vi "Dashboard Main.vi"() -> ()   [LabVIEW 2018]
uses:
  <vilib>/Utility/miscctls.llb/LVRowAndColumnTypeDef.ctl
  <vilib>/event_ctls.llb/eventvkey.ctl
  <vilib>/Utility/xml.llb/Read From XML File(array).vi
  <vilib>/Utility/xml.llb/Write to XML File(string).vi
  <vilib>/Rock Robotics/Network Tables/NT Read Boolean.vi
  <vilib>/Rock Robotics/Network Tables/NT Write Boolean.vi
  <vilib>/Rock Robotics/WPI/Dashboard/WPI_DashboardLogging Global.vi
  <vilib>/vision/NI_Vision_Development_Module.lvlib
panel:
  in  "TCP":refnum<k5>
  in  "Rec Mode":enum32{"Stop", "Record", "Playback"}(radio)
  out "Image Message":string="Timeout in Camera Communications"
  in  "Dashboard Tab":T1(tab)=enum."TeleOp"
  in  "CheckList":i32(listbox)
  in  "Driver Profile":u16(ring) items=["N/A"]
  in  "Camera Name":string(combo)="limelight"
  in  "Camera Settings":T2={"Frame Rate"=20, "Compression"=60, "Size"=1, "DB Camera Config"=FALSE} {"Size" items=["640x480", "320x240", "160x120"]}
  in  "Warning Time (s)":dbl=30.0
  out "Pressure_Leak":bool
  out "Ret_CARGO Right":bool
  out "Ret_HATCH Right":bool
  out "Ret_CARGO Left":bool
  out "Ret_HATCH Left":bool
  out "Ret_CARGO Center":bool
  out "Elevator_Motor_Failure_2":bool
  out "Elevator_Stall":bool
  out "Range_Color_Front-Right":u32(colorbox)
  in  "Right":bool
  in  "Reticule":T3(ring)
  in  "Save":bool
  in  "Up":bool
  in  "Down":bool
  in  "Left":bool
  out "Out_Of_Time":bool caption="Mode_Butterfly"
  out "Match Time(s)":sgl
  out "Intake_In":bool caption="Mode_Butterfly"
  in  "Climb_Safety":bool
  out "Master_Caution":bool caption="Mode_Butterfly"
  out "Climb_Sequence":string
  out "Range_to_Target (R)":i16(slide)=-100 scale=-10.0..-50.0
  out "Range_to_Target (L)":i16(slide)=-100 scale=-50.0..-10.0
  out "Tilt_Interlock":bool
  out "Battery_Critical":bool
  out "Battery_Voltage":dbl(slide) scale=11.0..13.0
  out "COM_Warning":bool
  out "Elevator_Moving":bool caption="Mode_Butterfly"
  out "Range_Color_Back":u32(colorbox)
  out "Range_Color_Front-Left":u32(colorbox)
  out "Range_Color_Right":u32(colorbox)
  out "Range_Color_Left":u32(colorbox)
  out "Hatch_Ship_Light":bool
  out "Hatch_Rocket_1_Light":bool
  out "Hatch_Ground_Light":bool
  out "Hatch_Feeder_Light":bool
  out "Hatch_Rocket_2_Light":bool
  out "Hatch_Rocket_3_Light":bool
  out "Pressure_Visualize":dbl(slide) scale=0.0..120.0
  out "Autopilot":bool caption="Mode_Butterfly"
  in  "Master_Safety_Override_1":bool
  in  "Master_Safety_Override_2":bool
  out "Climb_Light":bool
  out "At Climb_Height":bool caption="Mode_Butterfly"
  out "PTO_Engaged":bool caption="Mode_Butterfly"
  in  "Climb":bool
  out "Mode_Butterfly":bool
  out "Compressor_On":bool
  out "Hatch_Ejection_State":bool caption="Mode_Butterfly"
  out "Elevator_Brake_State":bool
  out "Mode_Shift":bool caption="Mode_Butterfly"
  out "Capture_Cargo":bool caption="Mode_Butterfly"
  out "Capture_Hatch":bool caption="Mode_Butterfly"
  in  "Hatch_Ground":bool
  in  "Hatch_Feeder":bool
  in  "Hatch_Rocket_2":bool
  in  "Hatch_Rocket_1":bool
  in  "Hatch_Ship":bool
  in  "Hatch_Rocket_3":bool
  out "Elevator_Stow_Light":bool
  in  "Elevator_Stow":bool
  out "Cargo_Ground_Light":bool
  out "Cargo_Feeder_Light":bool
  out "Cargo_Ship_Light":bool
  out "Cargo_Rocket_3_Light":bool
  in  "Cargo_Ground":bool
  in  "Cargo_Feeder":bool
  out "Cargo_Rocket_2_Light":bool
  out "Cargo_Rocket_1_Light":bool
  in  "Cargo_Ship":bool
  in  "Cargo_Rocket_1":bool
  in  "Cargo_Rocket_2":bool
  in  "Cargo_Rocket_3":bool
  out "State_Conflict":bool caption="Mode_Butterfly"
  out "Combined Camera Feed":T4(plugin-control)
  out "Elevator_Pos_Visual":dbl(slide) scale=34.5..89.0
  in  "Vision_Target_L_R":bool
  out "Elevator_Goal_Visual":dbl(slide) scale=34.5..89.0
  out "Elevator_Power":dbl(knob) scale=-1.0..1.0
  in  "Climb_Level":u8(slide)=1 scale=0.0..2.0
  out "E1 Warning":bool
  out "E2 Warning":bool
  out "E3 Warning":bool
  out "Elevator_3_Current":dbl format="%.1g"
  out "Elevator_2_Current":dbl format="%.1g"
  out "Elevator_1_Current":dbl format="%.1g"
  out "Slow_Loop":bool
  in  "Elevator_Kf_1":dbl(slide)=0.2 min=0.0 max=1.0 scale=0.0..1.0
  in  "Elevator_Kf_2":dbl(slide)=0.2 min=0.0 max=1.0 scale=0.0..1.0
  in  "Elevator_Kf_3":dbl(slide) min=0.0 max=1.0 scale=0.0..1.0
  in  "Select Auto":string(combo)="Select Autonomous ..."
  out "Camera Perf":string
  in  "Elevator_Kf_Climb":dbl(slide)=0.1 min=0.0 max=1.0 scale=0.0..1.0
  out "Control Loop Time (ms)":u32
  in  "Vacuum_Pump":dbl(slide)=0.6 min=0.0 max=1.0 scale=0.0..1.0
  out "Range_Right":dbl format="%.1g"
  in  "Elevator_Manual":bool
  in  "Drive_Encoder_Reset":bool
  out "Right_Drive_Pos":dbl
  out "Left_Drive_Pos":dbl
  out "Range_Left":dbl format="%.1g"
  out "Range_Front-Left":dbl format="%.1g"
  out "Range_Front-Right":dbl format="%.1g"
  out "Left_Drive_Vel":dbl format="%.1g"
  out "Right_Drive_Vel":dbl format="%.1g"
  out "Elevator_Pos":dbl format="%.1g"
  out "Range_Back":dbl
  out "Tank_Pressure":dbl format="%.1f"
  in  "Super_Test_Mode":bool
  out "Ground_Height":dbl format="%.1g"
  in  "Overclock":bool=TRUE
  in  "Reinit_Stow_Vacuum":bool
  in  "LimeLight_Override":bool
  out "Elevator_Encoder_Malfunction":bool
  out "Elevator_Motor_Failure":bool
  out "Robot_On_Ground":bool=TRUE
  out "Robot_Off_Ground":bool
  out "Check_Limit_Switch":bool
  in  "Tilt_Safety_Override":bool
  in  "Defense_Driving":bool
  out "Combined Error String":string
  out "NT Connection":bool
  out "Mode":T5(ring)=enum."Auto Disabled"
  in  "Test Slider":dbl(slide) scale=0.0..100.0 scale format="%#_3g"
  in  "On/Off":bool caption="Solenoid"
  in  "Test Name":u16(ring) items=["Select the test to run..."]
  in  "Test Tree":string(tree)
  in  "Motor":cluster{"Value":dbl, "Enable":bool} {"Value" scale=-1.0..1.0 scale format="%#_3g"}
  out "Progress":T6 {"Test Progress" scale=0.0..100.0}
  in  "Rev/Fwd":cluster{"Forward":bool, "Reverse":bool}
  in  "Test Ring":u16(ring) items=["Monochrome", "Color"]
  out "Cmd Status":string
  in  "Execute Command":bool
  in  "Command Params":string[][](table)
  in  "Command Selection":i32(listbox)
  out "Tree":string(tree)
  out "Background":bool
  # "Camera Selection"
  # "Match End Warning (s)"
  # "Camera Settings"
  # "89.0"
  # "11"
  # "13"
  # "120"
  # "0"
  # "Valkyrie"
  # "B"
  # "3"
  # "2"
  # "0"
  # "34.5"
  # "Control Loop (ms)"
  # "Elevator Feed Forward Coefficients"
  # "Drive Wheel Velocities (ft/s)"
  # "Manual Elevator Override"
  # "Tilt Interlock Off"
  # "Wide-Cam Override"
  # "Reinit.  Vacuum in Stow"
  # "Super Test Mode"
  # "Elevator Position (in)"
  # "Prox Sensors (in)"
  # "Auto Elevator"
  # "Safe"
  # "Vacuum \nPump Power"
  # "Normal"
  # "Normal"
  # "Safe"
  # "Stage 2"
  # "Stage 3"
  # "Climb"
  # "Ground Height (in)"
  # "Elevator Motor Currents (A)"
  # "On \nGround"
  # "Off\nGround"
  # "E1"
  # "E2"
  # "E3"
  # "Tank Pressure (psi)"
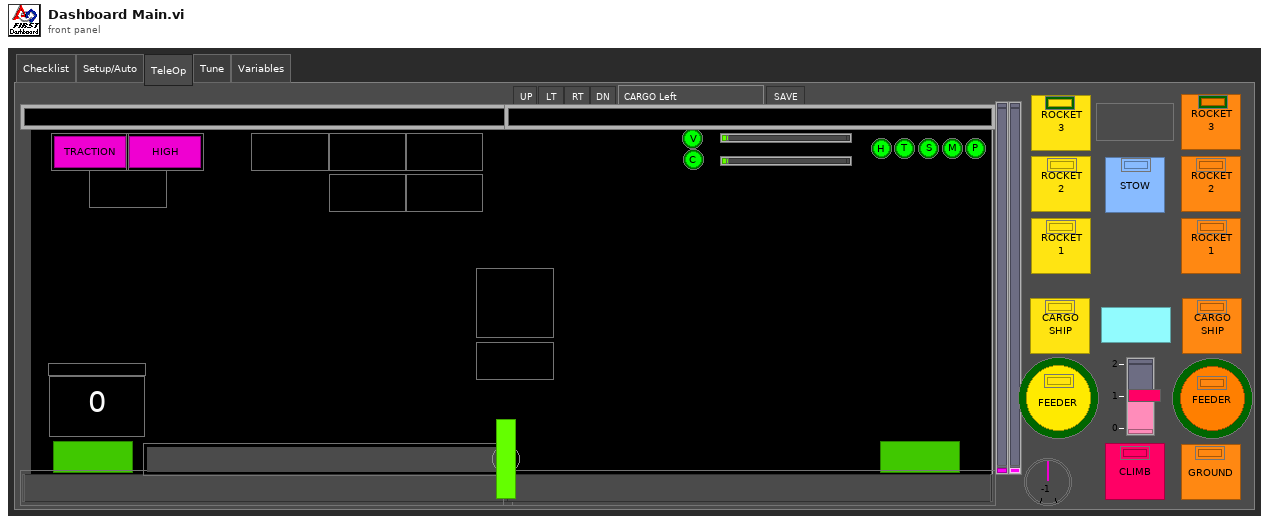
[diagram p1: front panel]
types:
  T1 = enum32{"Checklist", "Setup/Auto", "TeleOp", "Tune", "NT", "Test", "Commands", "Variables"}
  T2 = cluster{"Frame Rate":i32, "Compression":i32, "Size":u16, "DB Camera Config":bool}
  T3 = enum16{"CARGO Left", "CARGO Right", "HATCH Left", "HATCH Right", "CARGO Center"}
  T4 = typedef "IMAQ Image.ctl" = refnum<image>
  T5 = enum8{"Tele-Op Disabled", "Tele-Op Enabled", "Auto Disabled", "Auto Enabled", "Test Disabled", "Test Enabled", "Disconnected", "No Code", "E-Stop"}
  T6 = cluster{"Test Progress":u8, "Test Progress Text":string}
  T7 = cluster{"Save Path":path, "Interval (s)":dbl, "Keep":i32}
  T8 = enum32{"Drive", "Camera", "Basic", "Custom", "Test", "Commands", "Checklist", "Variables"}
  T9 = cluster{"IDs":cluster{"RPC field ID":u16, "Unique ID":u16}, "String":string}
  T10 = typedef "Image Type" = u32
  T11 = cluster{"Camera Name":string, string, "Saved DB Images Info":cluster{"Save Path":path, "Interval (s)":dbl, "Keep":i32}}
  T12 = cluster{"Ret_CARGO Left":refnum<vi>, "Ret_CARGO Right":refnum<vi>, "Ret_HATCH Left":refnum<vi>, "Ret_HATCH Right":refnum<vi>, "Ret_CARGO Center":refnum<vi>}
  T13 = enum32{"Checklist", "-", "TeleOp", "Tune", "NT", "Test", "Commands", "Variables"}
  T14 = cluster{"Error Strings":string, "Disable Counts":cluster{u16, u16}, "Rail Faults":cluster{u16, u16, u16}, "Robot IP":string, "DB Mode":u8, "Event Info":cluster{"Name":string, "Type":u8, "Number":u16, "Replay":u8}}
  T15 = cluster{"Storage":cluster{"Disk Free":u64, "RAM Block":u32, "RAM free":u32}, "CPU Utilization":cluster{"CPU % ISR":sgl, "CPU % Time Crit":sgl, "CPU % Timed Str":sgl, "CPU % High":sgl, "CPU % Above":sgl, "CPU % Normal":sgl, "CPU % Low":sgl}, "CAN":cluster{"% Bus Utilization":sgl, "Bus Off Cnt":u32, "TX_FIFO Full Cnt":u32, "Receive Error Cnt":u8, "Transmit Error Cnt":u8}, "HID":cluster{"HID Outputs":u32, "Rumble Low":u16, "Rumble High":u16}[]}
  T16 = cluster{"Status bits":cluster{"Test Mode":bool, "Autonomous":bool, "Enabled":bool, "Code Start":bool, "Brownout":bool, "Reserved 2":bool, "Reserved 3":bool, "E-Stop":bool}, "Code Trace":cluster{"Disabled":bool, "TeleOp":bool, "Auto":bool, "Test":bool}, "Controller Type":enum16{"unknown", "cRIO", "roboRio"}, "Code?":enum16{"unknown", "noCode", "code"}, "Battery V":dbl}
  T17 = cluster{"Control Bits":cluster{"TestMode":bool, "Autonomous":bool, "Enabled":bool, "FMS Present":bool, bool, bool, bool, "E-Stop":bool}, "Team Station ":u8, "Countdown":sgl, "Joystick Values":cluster{"Axes":dbl[], "Buttons":bool[], "POVs":i16[]}[]}
  T18 = cluster{"Operation":enum16{"Update", "Clear"}, "Color Box":u32}[]
  T19 = typedef "eventvkey.ctl" = enum16{"ASCII", "Enter", "Return", "Shift", "Ctrl", "Alt", "Cmd", "Opt", "Caps", "NumLock", "Clear", "Break", "Up", "Down", "Left", "Right", "Insert", "Delete", "Home", "End", "PageUp", "PageDown", "Escape", "Help", "Pause", "ScrollLock", "F1", "F2", "F3", "F4", "F5", "F6", "F7", "F8", "F9", "F10", "F11", "F12", "F13", "F14", "F15", "F16", "F17", "F18", "F19", "F20", "F21", "F22", "F23", "F24", "Play", "VolumeUp", "VolumeDown", "Mute", "Two Byte Char"}
  T20 = cluster{"Image Size":bool, "Image Type":bool, "Pixel Value":bool, "ROI Information":bool, "Zoom Factor":bool}
  T21 = cluster{"Operation":enum16{"Update", "Clear"}, "Color Box":u32}
  T22 = typedef "LVRowAndColumnTypeDef.ctl" = cluster{"Row":i32, "Column":i32}
  T23 = cluster{"Shift":bool, "Ctrl":bool, "Alt":bool, "Cmd":bool, "Opt":bool}
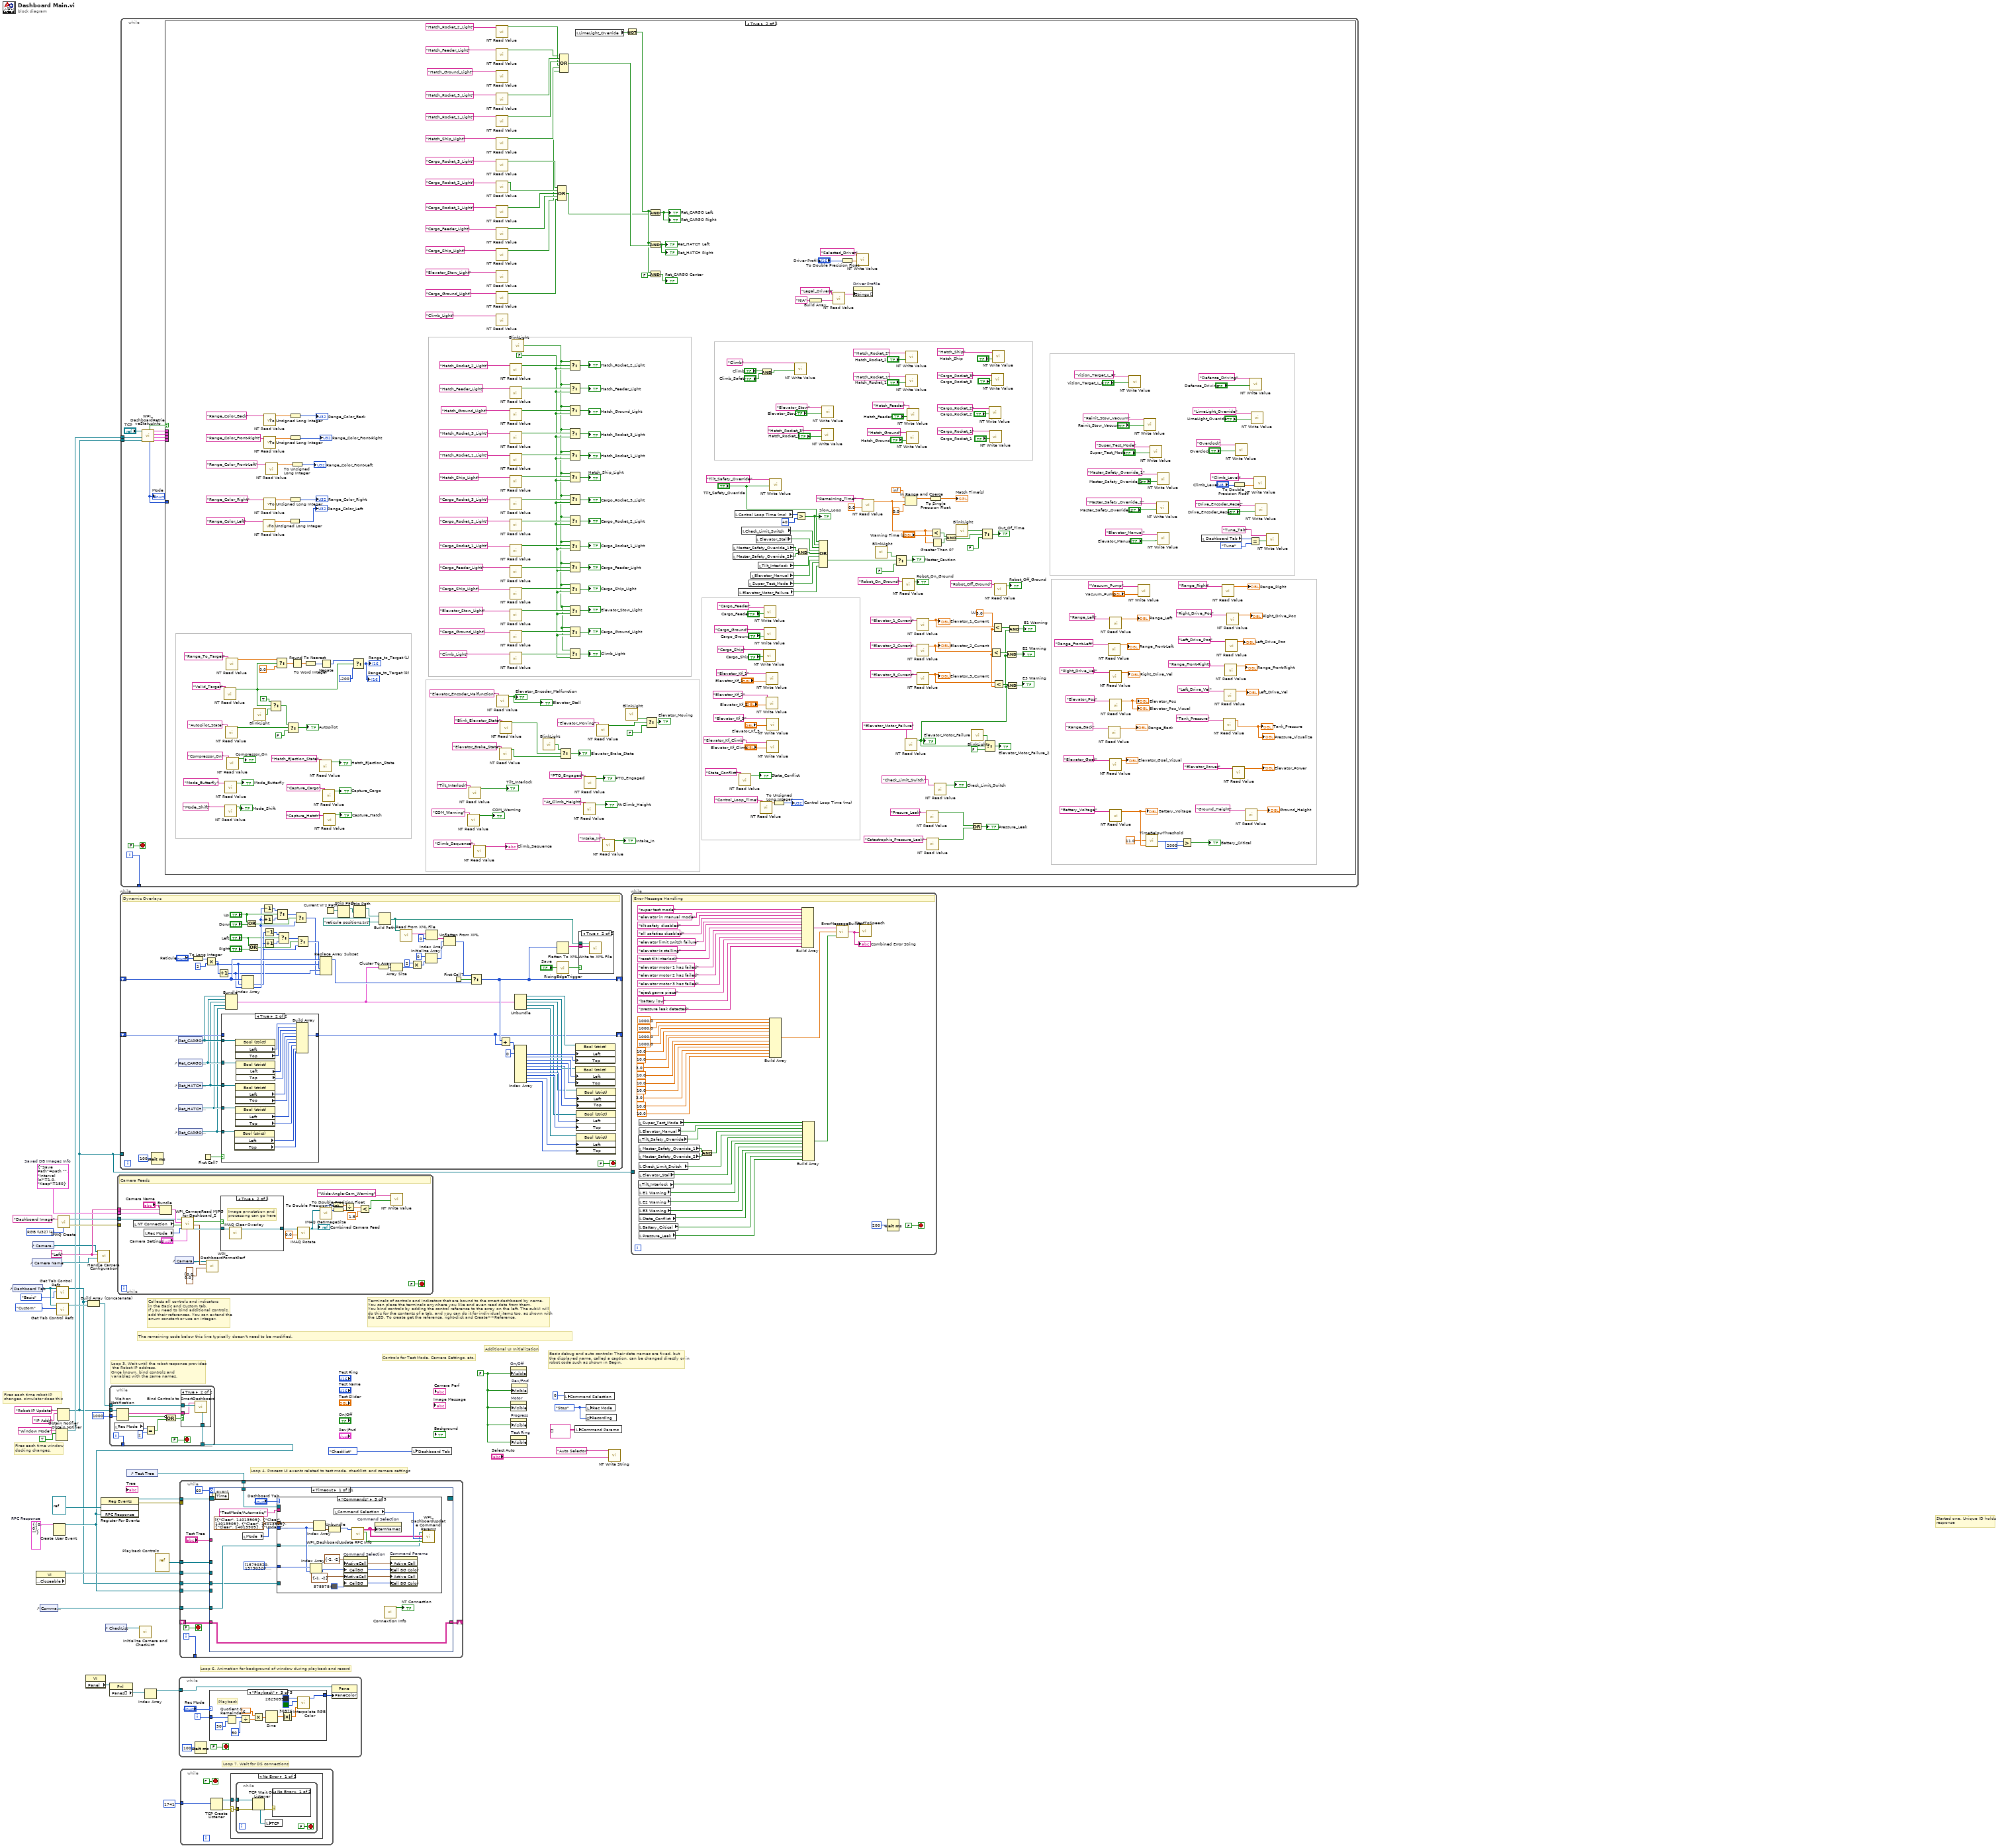
[diagram p0: block diagram]
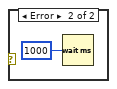
[diagram p4: hidden frame]
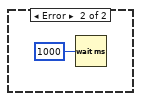
[diagram p5: hidden frame]
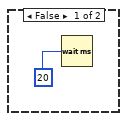
[diagram p6: hidden frame]
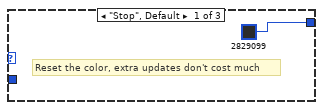
[diagram p7: hidden frame]
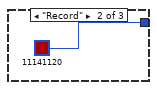
[diagram p8: hidden frame]
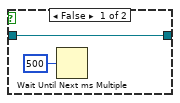
[diagram p10: hidden frame]
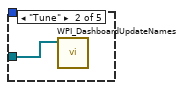
[diagram p12: hidden frame]
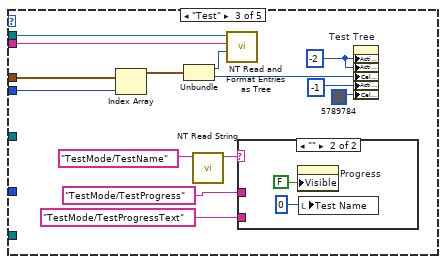
[diagram p13: hidden frame]
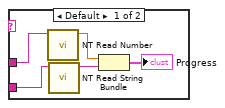
[diagram p14: hidden frame]
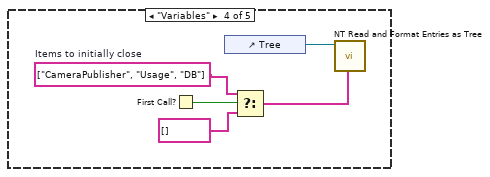
[diagram p15: hidden frame]
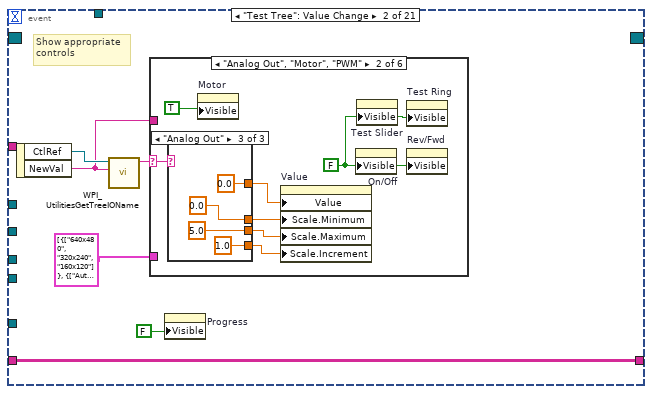
[diagram p16: hidden frame]
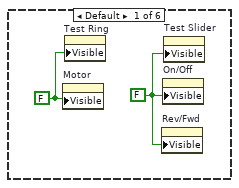
[diagram p17: hidden frame]
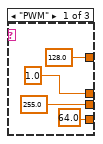
[diagram p18: hidden frame]
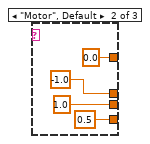
[diagram p19: hidden frame]
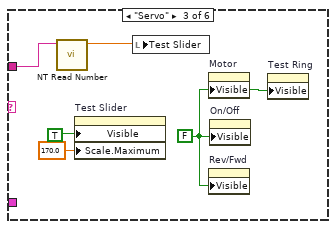
[diagram p20: hidden frame]
diagram:
  w4 = T7 {"Save Path"=path "", "Interval (s)"=1.0, "Keep"=180}  # Saved DB Images Info
  w3 = "Left"
  w15 = T9 {"IDs"={"RPC field ID"=0, "Unique ID"=0}, "String"=""}  # RPC Response
  w25 = enum32{"Stop", "Record", "Playback"}."Stop" ("Rec Mode")
  w19 = FALSE ("Visible")
  w42 = T10 4 items=["Grayscale (U8)", "Grayscale (I16)", "Grayscale (SGL)", "Complex (CSG)", "RGB (U32)", "HSL (U32)", "RGB (U64)"] ("Image Type")
  # "Started one, Unique ID holds\nresponse"
  # "Loop 7. Wait for DS connections"
  # "Basic debug and auto controls: Their data names are fixed, but\nthe displayed name, called a caption, can be changed directly or in\nrobot code such as shown in Begin."
  # "Controls for Test Mode, Camera Settings, etc."
  # "Additional UI Initialization"
  # "Loop 6. Animation for background of window during playback and record"
  # "Fires each time robot IP\nchanges, simulator does this"
  # "Fires each time window\ndocking changes."
  # "Collects all controls and indicators\nin the Basic and Custom tab.\nIf you need to bind additional controls,\nadd their references. You can extend the\nenum constant or use an integer."
  # "The remaining code below this line typically doesn't need to be modified."
  # "Loop 4. Process UI events related to test mode, checklist, and camera settings"
  # "Terminals of controls and indicators that are bound to the smart dashboard by name.\nYou can place the terminals anywhere you like and even read data from them.\nYou bind controls by adding the control reference to the array on the left. The subVI will\ndo this for the contents of a tab, and you can do it for individual items too, as shown with\nthe LED. To create get the reference, right-click and Create>>Reference."
  # "Loop 3. Wait until the robot response provides\n the Robot IP address.\nOnce known, bind controls and\nvariables with the same names."
  n1 = control-ref of="Dashboard Tab"() -> (w23:refnum<vi>)
  n2 = control-ref of="Camera Name"() -> (w10:refnum<vi>)
  n3 = control-ref of="Camera Settings"() -> (w2:refnum<vi>)
  n4 = property class="VI" props=["Front Panel.Closeable"]() -> (reference out=w24:refnum<vi>)  [unwired: 2 in, 2 out]
  n5 = control-ref of="Command Params"() -> (w11:refnum<vi>)
  n6 = Create User Event(user event datatype=w15) -> (user event=w12:refnum<user-event>)  [unwired: 1 in, 1 out]
  n7 = Obtain Notifier(name (unnamed)="Window Mode", notification data type=TRUE) -> (notifier out=w18:refnum<notifier>)  [unwired: 2 in, 2 out]
  n8 = call <vilib>:"Get Tab Control Refs.vi"("Page Index"=T8."Basic" ("Dashboard Tab"), "TabControl in"=w23) -> ("ControlsOnPage"=w9:refnum<vi>[])  [unwired: 9 in]
  n9 = call <vilib>:"Get Tab Control Refs.vi"("Page Index"=T8."Custom" ("Dashboard Tab"), "TabControl in"=w23) -> ("ControlsOnPage"=w22:refnum<vi>[])  [unwired: 9 in]
  n10 = Obtain Notifier(name (unnamed)="Robot IP Update", notification data type="IP Addr" ("name (unnamed)")) -> (notifier out=w1:refnum<notifier>)  [unwired: 2 in, 2 out]
  n11 = call "IMAQ Create"("Image Name"="Dashboard Image", "Image Type"=w42) -> ("New Image"=w40:T4, "error out"=w39:errorcluster)  [unwired: 2 in, 1 out]
  n12 = property class="VI"() -> ("Panel"=w32:refnum<vi>)  [unwired: 2 in, 2 out]
  n13 = Build Array (concatenate)(w9, w22) -> (w21:refnum<vi>[])
  n14 = call "Handle Camera Configuration.vi"("CameraNameRef"=w10, "Display Name"=w3, "ClusterRef"=w2) -> ()  [unwired: 9 in]
  n15 = register-events(refnum<vi> refnum, w12) -> (reference out=w29:refnum<event-registration>, error out=w28:errorcluster)  [unwired: 2 in]
  n16 = control-ref of="CheckList"() -> (w20:refnum<vi>)
  n17 = while {
    tunnel: w21 -> [w54]
    tunnel: w1 -> [w52]
    tunnel: [w50] -> _
    tunnel: u32 1000 ("milliseconds to wait") -> [w49]
    tunnel: w12 -> [w43]
    i -> [w50]
    stop <- FALSE stop-if-true
    n18 = local read "Rec Mode"() -> (w45:enum32{"Stop", "Record", "Playback"})
    n19 = Wait on Notification(notifier=w52, timeout in ms (-1)=w49) -> (notification=w51:string, timed out?=w47:bool)  [unwired: 2 in, 2 out]
    n20 = Equal?(x=w45, y=u16 2 ("Rec Mode")) -> (x = y?=w46:bool)
    n21 = Compound Arithmetic op=OR(invert w47, w46) -> (w48:bool)
    n22 = case shown="True" w48 {
      tunnel: w54 -> [_ w57]
      tunnel: w51 -> [_ w56]
      tunnel: w43 -> [_ w55]
      frame False {
      }
      frame True {
        n23 = call <vilib>:"Bind Controls to SmartDashboard.vi"("RPC ref"=w55, "Bound Control Refs"=w57, "Server IP Address"=w56) -> ()  [unwired: 9 in]
      }
    }
  }
  n24 = property class="Pnl"(reference=w32) -> ("Panes[]"=w33:refnum<vi>[])  [unwired: 1 in, 2 out]
  n25 = while {
    tunnel: w40 -> [w72]
    tunnel: w39 -> [_]
    tunnel: w4 -> [w77]
    tunnel: w3 -> [w75]
    stop <- FALSE stop-if-true
    # "Camera Feeds"
    n26 = local read "NT Connection"() -> (w78:bool)
    n27 = local read "Rec Mode"() -> (w79:enum32{"Stop", "Record", "Playback"})
    n28 = Bundle("Camera Name"="Camera Name", w75, "Saved DB Images Info"=w77) -> (w76:T11)  [unwired: 1 in]
    n29 = control-ref of="Camera Perf"() -> (w73:refnum<vi>)
    n30 = call <vilib>:"WPI_CameraRead MJPG for Dashboard_2.vi"("Camera Settings"="Camera Settings", "Rec Mode"=w79, "NT Connection"=w78, "Capture Info"=w76, "Image in"=w72) -> ("perf info"=w74:cluster{"Bandwidth (Mbps)":dbl, "fps":dbl}, "Active"=w80:bool, "Image\\ out"=w81:T4)  [unwired: 4 in]
    n31 = call <vilib>:"WPI_DashboardFormatPerf.vi"("Right Camera Perf"=cluster{"Bandwidth (Mbps)":dbl, "FPS":dbl} {"Bandwidth (Mbps)"=0.0, "FPS"=0.0}, "Performance"=w74, "String in"=w73) -> ()  [unwired: 9 in]
    n32 = case shown="True" w80 {
      tunnel: w81 -> [w83 w86]
      tunnel: [w83 w85] -> w71
      frame False {
        n33 = Wait Until Next ms Multiple(millisecond multiple=u32 500) -> ()  [unwired: 1 out]
      }
      frame True {
        # "Image annotation and\nprocessing can go here"
        n34 = call "IMAQ Clear Overlay"("Image"=w86) -> ("Image Out"=w85:T4)  [unwired: 2 in, 8 out]
      }
    }
    n35 = call "IMAQ Rotate"("Angle (degrees)"=sgl 0.0, "Image Src"=w71) -> ("Image Dst Out"=w68:T4)  [unwired: 8 in, 1 out]
    "Combined Camera Feed" <- w68
    n36 = call "IMAQ GetImageSize"("Image"=w68) -> ("Y Resolution"=w64:i32, "X Resolution"=w65:i32)  [unwired: 3 in, 1 out]
    n37 = To Double Precision Float(number=w65) -> (double precision float=w67:dbl)
    n38 = To Double Precision Float(number=w64) -> (double precision float=w66:dbl)
    n39 = Divide(x=w67, y=w66) -> (x/y=w63:dbl)
    n40 = Less?(x=w63, y=1.5) -> (x < y?=w61:bool)
    n41 = call-poly <vilib>:"NT Write Value.vi"("Boolean"=w61, "Name"="Wide-Angle-Cam_Warning") -> ()  [unwired: 9 in, 1 out]
  }
  n42 = while {
    shift-right: [w102] -> _
    shift-left: _ -> [w155]
    shift-right: [w106] -> _
    shift-left: _ -> [w145]
    tunnel: w1 -> [_]
    stop <- FALSE stop-if-true
    # "Dynamic Overlays"
    n43 = Wait (ms)(milliseconds to wait=u32 100) -> ()  [unwired: 1 out]
    n44 = control-ref of="Ret_CARGO Left"() -> (w111:refnum<vi>)
    n45 = control-ref of="Ret_CARGO Right"() -> (w110:refnum<vi>)
    n46 = control-ref of="Ret_HATCH Left"() -> (w96:refnum<vi>)
    n47 = control-ref of="Ret_HATCH Right"() -> (w95:refnum<vi>)
    n48 = control-ref of="Ret_CARGO Center"() -> (w92:refnum<vi>)
    n49 = To Long Integer(number="Reticule") -> (32bit integer=w136:i32)
    n50 = First Call?() -> (First Call?: T/F=w119:bool)
    n51 = Multiply(x=w136, y=2) -> (x*y=w135:i32)
    n52 = Increment(x=w135) -> (x+1=w114:i32)
    n53 = case shown="True" w119 {
      tunnel: w111 -> [_ w176]
      tunnel: [w160 w173] -> w102
      tunnel: w155 -> [w160 _]
      tunnel: w110 -> [_ w170]
      tunnel: w96 -> [_ w169]
      tunnel: w95 -> [_ w168]
      tunnel: w92 -> [_ w163]
      frame False {
      }
      frame True {
        n54 = property class="Bool (strict)"(reference=w163) -> ("Left"=w162:i32, "Top"=w161:i32)  [unwired: 1 in, 2 out]
        n55 = property class="Bool (strict)"(reference=w176) -> ("Left"=w175:i32, "Top"=w174:i32)  [unwired: 1 in, 2 out]
        n56 = property class="Bool (strict)"(reference=w169) -> ("Left"=w167:i32, "Top"=w166:i32)  [unwired: 1 in, 2 out]
        n57 = property class="Bool (strict)"(reference=w168) -> ("Left"=w165:i32, "Top"=w164:i32)  [unwired: 1 in, 2 out]
        n58 = property class="Bool (strict)"(reference=w170) -> ("Left"=w172:i32, "Top"=w171:i32)  [unwired: 1 in, 2 out]
        n59 = Build Array(w175, w174, w172, w171, w167, w166, w165, w164, w162, w161) -> (w173:i32[])
      }
    }
    n60 = Bundle("Ret_CARGO Left"=w111, "Ret_CARGO Right"=w110, "Ret_HATCH Left"=w96, "Ret_HATCH Right"=w95, "Ret_CARGO Center"=w92) -> (w104:T12)  [unwired: 1 in]
    n61 = Index Array(array=w145, index #1=w135, index #2=w114) -> (element #1=w139:i32, element #2=w147:i32)
    n62 = Or(x="Up", y="Down") -> (x .or. y?=w151:bool)
    n63 = Or(x="Left", y="Right") -> (x .or. y?=w141:bool)
    n64 = Decrement(x=w147) -> (x-1=w154:i32)
    n65 = Increment(x=w147) -> (x+1=w153:i32)
    n66 = Decrement(x=w139) -> (x-1=w144:i32)
    n67 = Increment(x=w139) -> (x+1=w143:i32)
    n68 = Select(t=w154, s="Up", f=w153) -> (s? t:f=w152:i32)
    n69 = Select(t=w144, s="Left", f=w143) -> (s? t:f=w142:i32)
    n70 = Select(t=w152, s=w151, f=w147) -> (s? t:f=w113:i32)
    n71 = Select(t=w142, s=w141, f=w139) -> (s? t:f=w140:i32)
    n72 = Replace Array Subset(array=w145, new element #1=w140, index #1=w135, new element #2=w113, index #2=w114) -> (w112:i32[])
    n73 = Current VI's Path() -> (path=w127:path)
    n74 = Strip Path(path=w127) -> (stripped path=w126:path)  [unwired: 1 out]
    n75 = Strip Path(path=w126) -> (stripped path=w125:path)  [unwired: 1 out]
    n76 = Cluster To Array(cluster=w104) -> (array=w109:refnum<vi>[])
    n77 = Build Path(base path=w125, name or relative path=path "reticule positions.txt" ("XML File Path")) -> (appended path=w124:path)
    n78 = Array Size(array=w109) -> (size(s)=w105:i32)
    n79 = call-poly <vilib>:"Read From XML File.vi"("XML File Path"=w124) -> ("XML Elements"=w123:string[])  [unwired: 8 in, 2 out]
    n80 = Multiply(x=2 ("dimension size"), y=w105) -> (x*y=w118:i32)
    n81 = Initialize Array(0, w118) -> (w88:i32[])
    n82 = Index Array(array=w123, index=0) -> (element=w121:string)
    n83 = Unflatten From XML(xml string=w121, type=w88) -> (value=w87:i32[])  [unwired: 1 in, 1 out]
    n84 = First Call?() -> (First Call?: T/F=w146:bool)
    n85 = Select(t=w87, s=w146, f=w112) -> (s? t:f=w106:i32[])
    n86 = Add(x=w106, y=w102) -> (x+y=w103:i32[])
    n87 = Unbundle(w104) -> ("Ret_CARGO Left"=w108:refnum<vi>, "Ret_CARGO Right"=w107:refnum<vi>, "Ret_HATCH Left"=w94:refnum<vi>, "Ret_HATCH Right"=w93:refnum<vi>, "Ret_CARGO Center"=w91:refnum<vi>)
    n88 = Index Array(array=w103, index #1=0 ("index")) -> (element #1=w133:i32, element #2=w132:i32, element #3=w116:i32, element #4=w115:i32, element #5=w100:i32, element #6=w99:i32, element #7=w98:i32, element #8=w97:i32, element #9=w90:i32, element #10=w89:i32)  [unwired: 9 in]
    n89 = Flatten To XML(anything=w106) -> (xml string=w131:string)
    n90 = call "RisingEdgeTrigger.vi"("Raw Signal"="Save") -> ("Trigger"=w130:bool)
    n91 = property class="Bool (strict)"(reference=w108, "Left"=w133, "Top"=w132) -> ()  [unwired: 1 in, 2 out]
    n92 = property class="Bool (strict)"(reference=w107, "Left"=w116, "Top"=w115) -> ()  [unwired: 1 in, 2 out]
    n93 = property class="Bool (strict)"(reference=w93, "Left"=w98, "Top"=w97) -> ()  [unwired: 1 in, 2 out]
    n94 = property class="Bool (strict)"(reference=w91, "Left"=w90, "Top"=w89) -> ()  [unwired: 1 in, 2 out]
    n95 = property class="Bool (strict)"(reference=w94, "Left"=w100, "Top"=w99) -> ()  [unwired: 1 in, 2 out]
    n96 = case shown="True" w130 {
      tunnel: w131 -> [_ w159]
      tunnel: w124 -> [_ w158]
      frame False {
      }
      frame True {
        n97 = call-poly <vilib>:"Write to XML File.vi"("XML Input"=w159, "XML File Path"=w158) -> ()  [unwired: 7 in, 3 out]
      }
    }
  }
  n98 = while {
    tunnel: [w186] -> _
    tunnel: w1 -> [w180]
    tunnel: w18 -> [w177]
    i -> [w186]
    stop <- FALSE stop-if-true
    n99 = call <vilib>:"WPI_DashboardRetrieveStatusInfo.vi"("Binding Refnum"=w180, "Window Mode Notifier"=w177, "TCP Cnx"="TCP") -> ("Power and Errors"=w181:T14, "Robot Metrics"=w184:T15, "Status Info"=w185:T16, "Control Info"=w182:T17, "Robot Mode"=w179:T5, "Process?"=w183:bool)  [unwired: 3 in]
    "Mode" <- w179
    n100 = case shown="True" w183 {
      tunnel: w185 -> [_ _]
      tunnel: w184 -> [_ _]
      tunnel: w182 -> [_ _]
      tunnel: w181 -> [_ _]
      tunnel: w179 -> [_ _]
      frame False {
        n101 = Wait (ms)(milliseconds to wait=u32 20) -> ()  [unwired: 1 out]
      }
      frame True {
        w220 = 5.0  # (A)
        w365 = FALSE ("f")
        n102 = call-poly <vilib>:"NT Read Value.vi"("Name"="Valid_Target") -> ("Boolean"=w337:bool)  [unwired: 9 in, 1 out]
        n103 = call-poly <vilib>:"NT Read Value.vi"("Name"="Mode_Shift") -> ("Boolean"=→"Mode_Shift":bool)  [unwired: 9 in, 1 out]
        n104 = call-poly <vilib>:"NT Read Value.vi"("Name"="Mode_Butterfly") -> ("Boolean"=→"Mode_Butterfly":bool)  [unwired: 9 in, 1 out]
        n105 = call-poly <vilib>:"NT Read Value.vi"("Name"="Autopilot_State") -> ("Boolean"=w351:bool)  [unwired: 9 in, 1 out]
        n106 = call-poly <vilib>:"NT Read Value.vi"("Name"="Range_To_Target") -> ("Numeric"=w344:dbl)  [unwired: 9 in, 1 out]
        n107 = call-poly <vilib>:"NT Read Value.vi"("Name"="Compressor_On") -> ("Boolean"=→"Compressor_On":bool)  [unwired: 9 in, 1 out]
        n108 = call "BlinkLight.vi"() -> ("Blinked"=w346:bool)  [unwired: 1 in]
        n109 = call-poly <vilib>:"NT Read Value.vi"("Name"="Range_Color_Left") -> ("Numeric"=w502:dbl)  [unwired: 9 in, 1 out]
        n110 = call-poly <vilib>:"NT Read Value.vi"("Name"="Range_Color_Back") -> ("Numeric"=w508:dbl)  [unwired: 9 in, 1 out]
        n111 = call-poly <vilib>:"NT Read Value.vi"("Name"="Range_Color_Front-Right") -> ("Numeric"=w506:dbl)  [unwired: 9 in, 1 out]
        n112 = call-poly <vilib>:"NT Read Value.vi"("Name"="Range_Color_Right") -> ("Numeric"=w504:dbl)  [unwired: 9 in, 1 out]
        n113 = call-poly <vilib>:"NT Read Value.vi"("Name"="Range_Color_Front-Left") -> ("Numeric"=w456:dbl)  [unwired: 9 in, 1 out]
        n114 = Select(t=TRUE, s=w337, f=w346) -> (s? t:f=w349:bool)
        n115 = Select(t=w344, s=w337, f=0.0) -> (s? t:f=w342:dbl)
        n116 = Select(t=w349, s=w351, f=FALSE) -> (s? t:f=→"Autopilot":bool)
        n117 = To Unsigned Long Integer(number=w502) -> (unsigned 32bit integer=→"Range_Color_Left":u32)
        n118 = To Unsigned Long Integer(number=w508) -> (unsigned 32bit integer=→"Range_Color_Back":u32)
        n119 = To Unsigned Long Integer(number=w506) -> (unsigned 32bit integer=→"Range_Color_Front-Right":u32)
        n120 = To Unsigned Long Integer(number=w504) -> (unsigned 32bit integer=→"Range_Color_Right":u32)
        n121 = To Unsigned Long Integer(number=w456) -> (unsigned 32bit integer=→"Range_Color_Front-Left":u32)
        n122 = Round To Nearest(number=w342) -> (nearest integer value=w341:dbl)
        n123 = To Word Integer(number=w341) -> (16bit integer=w340:i16)
        n124 = call-poly <vilib>:"NT Read Value.vi"("Name"="Hatch_Ejection_State") -> ("Boolean"=→"Hatch_Ejection_State":bool)  [unwired: 9 in, 1 out]
        n125 = Negate(x=w340) -> (-x=w338:i16)
        n126 = call-poly <vilib>:"NT Read Value.vi"("Name"="Capture_Cargo") -> ("Boolean"=→"Capture_Cargo":bool)  [unwired: 9 in, 1 out]
        n127 = call-poly <vilib>:"NT Read Value.vi"("Name"="Capture_Hatch") -> ("Boolean"=→"Capture_Hatch":bool)  [unwired: 9 in, 1 out]
        n128 = Select(t=w338, s=w337, f=i16 -200) -> (s? t:f=→"Range_to_Target (L)" →"Range_to_Target (R)":i16)
        n129 = call-poly <vilib>:"NT Read Value.vi"("Name"="COM_Warning") -> ("Boolean"=→"COM_Warning":bool)  [unwired: 9 in, 1 out]
        n130 = call-poly <vilib>:"NT Read Value.vi"("Name"="Tilt_Interlock") -> ("Boolean"=→"Tilt_Interlock":bool)  [unwired: 9 in, 1 out]
        n131 = call-poly <vilib>:"NT Read Value.vi"("Name"="Climb_Sequence") -> ("String"=→"Climb_Sequence":string)  [unwired: 9 in, 1 out]
        n132 = call-poly <vilib>:"NT Read Value.vi"("Name"="Hatch_Rocket_2_Light") -> ("Boolean"=w260:bool)  [unwired: 9 in, 1 out]
        n133 = call-poly <vilib>:"NT Read Value.vi"("Name"="Hatch_Feeder_Light") -> ("Boolean"=w258:bool)  [unwired: 9 in, 1 out]
        n134 = call-poly <vilib>:"NT Read Value.vi"("Name"="Hatch_Ground_Light") -> ()  [unwired: 9 in, 2 out]
        n135 = call-poly <vilib>:"NT Read Value.vi"("Name"="Hatch_Rocket_3_Light") -> ("Boolean"=w262:bool)  [unwired: 9 in, 1 out]
        n136 = call-poly <vilib>:"NT Read Value.vi"("Name"="Hatch_Rocket_1_Light") -> ("Boolean"=w261:bool)  [unwired: 9 in, 1 out]
        n137 = call-poly <vilib>:"NT Read Value.vi"("Name"="Hatch_Ship_Light") -> ("Boolean"=w259:bool)  [unwired: 9 in, 1 out]
        n138 = call-poly <vilib>:"NT Read Value.vi"("Name"="Cargo_Rocket_3_Light") -> ("Boolean"=w243:bool)  [unwired: 9 in, 1 out]
        n139 = call-poly <vilib>:"NT Read Value.vi"("Name"="Cargo_Rocket_2_Light") -> ("Boolean"=w242:bool)  [unwired: 9 in, 1 out]
        n140 = call-poly <vilib>:"NT Read Value.vi"("Name"="Cargo_Rocket_1_Light") -> ("Boolean"=w241:bool)  [unwired: 9 in, 1 out]
        n141 = call-poly <vilib>:"NT Read Value.vi"("Name"="Cargo_Feeder_Light") -> ("Boolean"=w240:bool)  [unwired: 9 in, 1 out]
        n142 = call-poly <vilib>:"NT Read Value.vi"("Name"="Cargo_Ship_Light") -> ("Boolean"=w206:bool)  [unwired: 9 in, 1 out]
        n143 = call-poly <vilib>:"NT Read Value.vi"("Name"="Elevator_Stow_Light") -> ()  [unwired: 9 in, 2 out]
        n144 = call-poly <vilib>:"NT Read Value.vi"("Name"="Cargo_Ground_Light") -> ("Boolean"=w205:bool)  [unwired: 9 in, 1 out]
        n145 = call-poly <vilib>:"NT Read Value.vi"("Name"="Climb_Light") -> ()  [unwired: 9 in, 2 out]
        n146 = call-poly <vilib>:"NT Read Value.vi"("Name"="Elevator_Encoder_Malfunction") -> ("Boolean"=→"Elevator_Encoder_Malfunction" →"Elevator_Stall":bool)  [unwired: 9 in, 1 out]
        n147 = call-poly <vilib>:"NT Read Value.vi"("Name"="Elevator_Brake_State") -> ("Boolean"=w361:bool)  [unwired: 9 in, 1 out]
        n148 = call-poly <vilib>:"NT Read Value.vi"("Name"="Blink_Elevator_State") -> ("Boolean"=w360:bool)  [unwired: 9 in, 1 out]
        n149 = call-poly <vilib>:"NT Read Value.vi"("Name"="Hatch_Rocket_2_Light") -> ("Boolean"=w415:bool)  [unwired: 9 in, 1 out]
        n150 = call-poly <vilib>:"NT Read Value.vi"("Name"="Hatch_Feeder_Light") -> ("Boolean"=w413:bool)  [unwired: 9 in, 1 out]
        n151 = call-poly <vilib>:"NT Read Value.vi"("Name"="Hatch_Ground_Light") -> ("Boolean"=w412:bool)  [unwired: 9 in, 1 out]
        n152 = call-poly <vilib>:"NT Read Value.vi"("Name"="Hatch_Rocket_3_Light") -> ("Boolean"=w416:bool)  [unwired: 9 in, 1 out]
        n153 = call-poly <vilib>:"NT Read Value.vi"("Name"="Hatch_Rocket_1_Light") -> ("Boolean"=w414:bool)  [unwired: 9 in, 1 out]
        n154 = call-poly <vilib>:"NT Read Value.vi"("Name"="Hatch_Ship_Light") -> ("Boolean"=w411:bool)  [unwired: 9 in, 1 out]
        n155 = call-poly <vilib>:"NT Read Value.vi"("Name"="Cargo_Rocket_3_Light") -> ("Boolean"=w426:bool)  [unwired: 9 in, 1 out]
        n156 = call-poly <vilib>:"NT Read Value.vi"("Name"="Cargo_Rocket_2_Light") -> ("Boolean"=w425:bool)  [unwired: 9 in, 1 out]
        n157 = call-poly <vilib>:"NT Read Value.vi"("Name"="Cargo_Rocket_1_Light") -> ("Boolean"=w424:bool)  [unwired: 9 in, 1 out]
        n158 = call-poly <vilib>:"NT Read Value.vi"("Name"="Cargo_Feeder_Light") -> ("Boolean"=w423:bool)  [unwired: 9 in, 1 out]
        n159 = call-poly <vilib>:"NT Read Value.vi"("Name"="Cargo_Ship_Light") -> ("Boolean"=w429:bool)  [unwired: 9 in, 1 out]
        n160 = call-poly <vilib>:"NT Read Value.vi"("Name"="Elevator_Stow_Light") -> ("Boolean"=w379:bool)  [unwired: 9 in, 1 out]
        n161 = call-poly <vilib>:"NT Read Value.vi"("Name"="Cargo_Ground_Light") -> ("Boolean"=w427:bool)  [unwired: 9 in, 1 out]
        n162 = call-poly <vilib>:"NT Read Value.vi"("Name"="Climb_Light") -> ("Boolean"=w428:bool)  [unwired: 9 in, 1 out]
        n163 = call "BlinkLight.vi"() -> ("Blinked"=w364:bool)  [unwired: 1 in]
        n164 = call "BlinkLight.vi"() -> ("Blinked"=w359:bool)  [unwired: 1 in]
        n165 = Compound Arithmetic op=OR(w243, w242, w241, w240, w205) -> (w238:bool)
        n166 = Compound Arithmetic op=OR(w258, w262, w261, w260, w259, w206) -> (w257:bool)
        n167 = Select(t=w359, s=w360, f=w361) -> (s? t:f=→"Elevator_Brake_State":bool)
        n168 = Select(t=w364, s=w415, f=w365) -> (s? t:f=→"Hatch_Rocket_2_Light":bool)
        n169 = Select(t=w364, s=w413, f=w365) -> (s? t:f=→"Hatch_Feeder_Light":bool)
        n170 = Select(t=w364, s=w412, f=w365) -> (s? t:f=→"Hatch_Ground_Light":bool)
        n171 = Select(t=w364, s=w416, f=w365) -> (s? t:f=→"Hatch_Rocket_3_Light":bool)
        n172 = Select(t=w364, s=w414, f=w365) -> (s? t:f=→"Hatch_Rocket_1_Light":bool)
        n173 = Select(t=w364, s=w411, f=w365) -> (s? t:f=→"Hatch_Ship_Light":bool)
        n174 = Select(t=w364, s=w426, f=w365) -> (s? t:f=→"Cargo_Rocket_3_Light":bool)
        n175 = Select(t=w364, s=w425, f=w365) -> (s? t:f=→"Cargo_Rocket_2_Light":bool)
        n176 = Select(t=w364, s=w424, f=w365) -> (s? t:f=→"Cargo_Rocket_1_Light":bool)
        n177 = Select(t=w364, s=w423, f=w365) -> (s? t:f=→"Cargo_Feeder_Light":bool)
        n178 = Select(t=w364, s=w429, f=w365) -> (s? t:f=→"Cargo_Ship_Light":bool)
        n179 = Select(t=w364, s=w379, f=w365) -> (s? t:f=→"Elevator_Stow_Light":bool)
        n180 = Select(t=w364, s=w427, f=w365) -> (s? t:f=→"Cargo_Ground_Light":bool)
        n181 = Select(t=w364, s=w428, f=w365) -> (s? t:f=→"Climb_Light":bool)
        n182 = local read "LimeLight_Override"() -> (w265:bool)
        n183 = call-poly <vilib>:"NT Read Value.vi"("Name"="At_Climb_Height") -> ("Boolean"=→"At Climb_Height":bool)  [unwired: 9 in, 1 out]
        n184 = call-poly <vilib>:"NT Read Value.vi"("Name"="PTO_Engaged") -> ("Boolean"=→"PTO_Engaged":bool)  [unwired: 9 in, 1 out]
        n185 = call-poly <vilib>:"NT Read Value.vi"("Name"="Elevator_Moving") -> ("Boolean"=w328:bool)  [unwired: 9 in, 1 out]
        n186 = call-poly <vilib>:"NT Read Value.vi"("Name"="Intake_In") -> ("Boolean"=→"Intake_In":bool)  [unwired: 9 in, 1 out]
        n187 = call "BlinkLight.vi"() -> ("Blinked"=w329:bool)  [unwired: 1 in]
        n188 = Not(x=w265) -> (.not. x?=w244:bool)
        n189 = Select(t=w329, s=w328, f=FALSE) -> (s? t:f=→"Elevator_Moving":bool)
        n190 = Compound Arithmetic op=AND(w244, w238) -> (→"Ret_CARGO Left" →"Ret_CARGO Right":bool)
        n191 = Compound Arithmetic op=AND(w244, w257) -> (→"Ret_HATCH Left" →"Ret_HATCH Right":bool)
        n192 = Compound Arithmetic op=AND(w244, FALSE ("value")) -> (→"Ret_CARGO Center":bool)
        n193 = local read "Master_Safety_Override_1"() -> (w307:bool)
        n194 = local read "Master_Safety_Override_2"() -> (w306:bool)
        n195 = local read "Control Loop Time (ms)"() -> (w301:u32)
        n196 = local read "Elevator_Motor_Failure"() -> (w237:bool)
        n197 = call-poly <vilib>:"NT Read Value.vi"("Name"="State_Conflict") -> ("Boolean"=→"State_Conflict":bool)  [unwired: 9 in, 1 out]
        n198 = local read "Check_Limit_Switch"() -> (w211:bool)
        n199 = local read "Super_Test_Mode"() -> (w302:bool)
        n200 = local read "Elevator_Manual"() -> (w303:bool)
        n201 = local read "Elevator_Stall"() -> (w305:bool)
        n202 = local read "Tilt_Interlock"() -> (w304:bool)
        n203 = call-poly <vilib>:"NT Read Value.vi"("Name"="Control_Loop_Time") -> ("Numeric"=w447:dbl)  [unwired: 9 in, 1 out]
        n204 = And(x="Climb", y="Climb_Safety") -> (x .and. y?=w334:bool)
        n205 = call-poly <vilib>:"NT Write Value.vi"("Boolean"="Cargo_Ship", "Name"="Cargo_Ship") -> ()  [unwired: 9 in, 1 out]
        n206 = call-poly <vilib>:"NT Write Value.vi"("Boolean"="Cargo_Feeder", "Name"="Cargo_Feeder") -> ()  [unwired: 9 in, 1 out]
        n207 = call-poly <vilib>:"NT Write Value.vi"("Boolean"="Cargo_Ground", "Name"="Cargo_Ground") -> ()  [unwired: 9 in, 1 out]
        n208 = call-poly <vilib>:"NT Write Value.vi"("Numeric"="Elevator_Kf_2", "Name"="Elevator_Kf_2") -> ()  [unwired: 9 in, 1 out]
        n209 = call-poly <vilib>:"NT Write Value.vi"("Numeric"="Elevator_Kf_1", "Name"="Elevator_Kf_1") -> ()  [unwired: 9 in, 1 out]
        n210 = call-poly <vilib>:"NT Write Value.vi"("Numeric"="Elevator_Kf_3", "Name"="Elevator_Kf_3") -> ()  [unwired: 9 in, 1 out]
        n211 = call-poly <vilib>:"NT Write Value.vi"("Numeric"="Elevator_Kf_Climb", "Name"="Elevator_Kf_Climb") -> ()  [unwired: 9 in, 1 out]
        n212 = call-poly <vilib>:"NT Write Value.vi"("Boolean"="Tilt_Safety_Override", "Name"="Tilt_Safety_Override") -> ()  [unwired: 9 in, 1 out]
        n213 = To Unsigned Long Integer(number=w447) -> (unsigned 32bit integer=→"Control Loop Time (ms)":u32)
        n214 = call-poly <vilib>:"NT Write Value.vi"("Boolean"=w334, "Name"="Climb") -> ()  [unwired: 9 in, 1 out]
        n215 = Greater?(x=w301, y=u32 40) -> (0:w212:bool)
        "Slow_Loop" <- w212
        n216 = And(x=w307, y=w306) -> (x .and. y?=w308:bool)
        n217 = Build Array("N/A") -> (w199:string[])
        n218 = Compound Arithmetic op=OR("Tilt_Safety_Override", w212, w211, w305, w308, w304, w303, w302, w237) -> (w226:bool)
        n219 = call-poly <vilib>:"NT Write Value.vi"("Boolean"="Hatch_Rocket_3", "Name"="Hatch_Rocket_3") -> ()  [unwired: 9 in, 1 out]
        n220 = call-poly <vilib>:"NT Write Value.vi"("Boolean"="Elevator_Stow", "Name"="Elevator_Stow") -> ()  [unwired: 9 in, 1 out]
        n221 = call-poly <vilib>:"NT Read Value.vi"("Default Value"=w199, "Name"="Legal_Drivers") -> ("String Array"=w201:string[])  [unwired: 8 in, 1 out]
        n222 = To Double Precision Float(number="Driver Profile") -> (double precision float=w204:dbl)
        n223 = property on="Driver Profile" class="Ring (strict)"("Strings []"=w201) -> ()  [unwired: 2 in, 2 out]
        n224 = call-poly <vilib>:"NT Write Value.vi"("Numeric"=w204, "Name"="Selected_Driver") -> ()  [unwired: 9 in, 1 out]
        n225 = call-poly <vilib>:"NT Read Value.vi"("Default Value"=0.0, "Name"="Remaining_Time") -> ("Numeric"=w280:dbl)  [unwired: 8 in, 1 out]
        n226 = call "BlinkLight.vi"() -> ("Blinked"=w311:bool)  [unwired: 1 in]
        n227 = Select(t=w311, s=w226, f=FALSE) -> (s? t:f=→"Master_Caution":bool)
        n228 = call-poly <vilib>:"NT Read Value.vi"("Name"="Robot_On_Ground") -> ("Boolean"=→"Robot_On_Ground":bool)  [unwired: 9 in, 1 out]
        n229 = call-poly <vilib>:"NT Read Value.vi"("Name"="Elevator_Motor_Failure") -> ("Boolean"=w213:bool)  [unwired: 9 in, 1 out]
        "Elevator_Motor_Failure" <- w213
        n230 = In Range and Coerce(upper limit=inf, x=w280, lower limit=0.0) -> (coerced(x)=w283:dbl)  [unwired: 1 out]
        n231 = call-poly <vilib>:"NT Write Value.vi"("Boolean"="Hatch_Rocket_2", "Name"="Hatch_Rocket_2") -> ()  [unwired: 9 in, 1 out]
        n232 = call-poly <vilib>:"NT Write Value.vi"("Boolean"="Hatch_Rocket_1", "Name"="Hatch_Rocket_1") -> ()  [unwired: 9 in, 1 out]
        n233 = call-poly <vilib>:"NT Write Value.vi"("Boolean"="Hatch_Ground", "Name"="Hatch_Ground") -> ()  [unwired: 9 in, 1 out]
        n234 = call-poly <vilib>:"NT Write Value.vi"("Boolean"="Hatch_Feeder", "Name"="Hatch_Feeder") -> ()  [unwired: 9 in, 1 out]
        n235 = call-poly <vilib>:"NT Read Value.vi"("Name"="Elevator_1_Current") -> ("Numeric"=w223:dbl)  [unwired: 9 in, 1 out]
        "Elevator_1_Current" <- w223
        n236 = call-poly <vilib>:"NT Read Value.vi"("Name"="Elevator_2_Current") -> ("Numeric"=w222:dbl)  [unwired: 9 in, 1 out]
        "Elevator_2_Current" <- w222
        n237 = call-poly <vilib>:"NT Read Value.vi"("Name"="Elevator_3_Current") -> ("Numeric"=w221:dbl)  [unwired: 9 in, 1 out]
        "Elevator_3_Current" <- w221
        n238 = call-poly <vilib>:"NT Read Value.vi"("Name"="Presure_Leak") -> ("Boolean"=w190:bool)  [unwired: 9 in, 1 out]
        n239 = call-poly <vilib>:"NT Read Value.vi"("Name"="Catastrophic_Pressure_Leak") -> ("Boolean"=w189:bool)  [unwired: 9 in, 1 out]
        n240 = To Single Precision Float(number=w283) -> (single precision float=→"Match Time(s)":sgl)
        n241 = Less?(x=w280, y="Warning Time (s)") -> (x < y?=w286:bool)
        n242 = Greater Than 0?(x=w280) -> (x > 0?=w285:bool)
        n243 = call-poly <vilib>:"NT Read Value.vi"("Name"="Check_Limit_Switch") -> ("Boolean"=→"Check_Limit_Switch":bool)  [unwired: 9 in, 1 out]
        n244 = And(x=w286, y=w285) -> (x .and. y?=w284:bool)
        n245 = call "BlinkLight.vi"() -> ("Blinked"=w288:bool)  [unwired: 1 in]
        n246 = Or(x=w190, y=w189) -> (x .or. y?=→"Pressure_Leak":bool)
        n247 = call "BlinkLight.vi"() -> ("Blinked"=w248:bool)  [unwired: 1 in]
        n248 = Select(t=w288, s=w284, f=FALSE) -> (s? t:f=→"Out_Of_Time":bool)
        n249 = Select(t=w248, s=w213, f=FALSE) -> (s? t:f=→"Elevator_Motor_Failure_2":bool)
        n250 = call-poly <vilib>:"NT Write Value.vi"("Boolean"="Cargo_Rocket_2", "Name"="Cargo_Rocket_2") -> ()  [unwired: 9 in, 1 out]
        n251 = call-poly <vilib>:"NT Write Value.vi"("Boolean"="Cargo_Rocket_1", "Name"="Cargo_Rocket_1") -> ()  [unwired: 9 in, 1 out]
        n252 = Less?(x=w222, y=w220) -> (x < y?=w218:bool)
        n253 = call-poly <vilib>:"NT Write Value.vi"("Boolean"="Cargo_Rocket_3", "Name"="Cargo_Rocket_3") -> ()  [unwired: 9 in, 1 out]
        n254 = Less?(x=w223, y=w220) -> (x < y?=w219:bool)
        n255 = call-poly <vilib>:"NT Write Value.vi"("Boolean"="Hatch_Ship", "Name"="Hatch_Ship") -> ()  [unwired: 9 in, 1 out]
        n256 = Less?(x=w221, y=w220) -> (x < y?=w217:bool)
        n257 = call-poly <vilib>:"NT Read Value.vi"("Name"="Robot_Off_Ground") -> ("Boolean"=→"Robot_Off_Ground":bool)  [unwired: 9 in, 1 out]
        n258 = Compound Arithmetic op=AND(w218, w213) -> (→"E2 Warning":bool)
        n259 = Compound Arithmetic op=AND(w217, w213) -> (→"E3 Warning":bool)
        n260 = Compound Arithmetic op=AND(w219, w213) -> (→"E1 Warning":bool)
        n261 = call-poly <vilib>:"NT Read Value.vi"("Name"="Range_Front-Left") -> ("Numeric"=→"Range_Front-Left":dbl)  [unwired: 9 in, 1 out]
        n262 = call-poly <vilib>:"NT Read Value.vi"("Name"="Range_Back") -> ("Numeric"=→"Range_Back":dbl)  [unwired: 9 in, 1 out]
        n263 = call-poly <vilib>:"NT Read Value.vi"("Name"="Right_Drive_Vel") -> ("Numeric"=→"Right_Drive_Vel":dbl)  [unwired: 9 in, 1 out]
        n264 = call-poly <vilib>:"NT Read Value.vi"("Name"="Elevator_Goal") -> ("Numeric"=→"Elevator_Goal_Visual":dbl)  [unwired: 9 in, 1 out]
        n265 = call-poly <vilib>:"NT Read Value.vi"("Name"="Range_Left") -> ("Numeric"=→"Range_Left":dbl)  [unwired: 9 in, 1 out]
        n266 = call-poly <vilib>:"NT Read Value.vi"("Name"="Elevator_Pos") -> ("Numeric"=→"Elevator_Pos" →"Elevator_Pos_Visual":dbl)  [unwired: 9 in, 1 out]
        n267 = call-poly <vilib>:"NT Read Value.vi"("Name"="Battery_Voltage") -> ("Numeric"=w230:dbl)  [unwired: 9 in, 1 out]
        "Battery_Voltage" <- w230
        n268 = call-poly <vilib>:"NT Write Value.vi"("Boolean"="Vision_Target_L_R", "Name"="Vision_Target_L_R") -> ()  [unwired: 9 in, 1 out]
        n269 = call-poly <vilib>:"NT Write Value.vi"("Numeric"="Vacuum_Pump", "Name"="Vacuum_Pump") -> ()  [unwired: 9 in, 1 out]
        n270 = call-poly <vilib>:"NT Write Value.vi"("Boolean"="Reinit_Stow_Vacuum", "Name"="Reinit_Stow_Vacuum") -> ()  [unwired: 9 in, 1 out]
        n271 = call "TimeBelowThreshold.vi"("Current Value"=w230, "Threshold"=11.0 ("y")) -> ("Time Below"=w228:u32)  [unwired: 3 in]
        n272 = call-poly <vilib>:"NT Write Value.vi"("Boolean"="Super_Test_Mode", "Name"="Super_Test_Mode") -> ()  [unwired: 9 in, 1 out]
        n273 = call-poly <vilib>:"NT Write Value.vi"("Boolean"="Master_Safety_Override_2", "Name"="Master_Safety_Override_2") -> ()  [unwired: 9 in, 1 out]
        n274 = call-poly <vilib>:"NT Write Value.vi"("Boolean"="Master_Safety_Override_1", "Name"="Master_Safety_Override_1") -> ()  [unwired: 9 in, 1 out]
        n275 = call-poly <vilib>:"NT Write Value.vi"("Boolean"="Elevator_Manual", "Name"="Elevator_Manual") -> ()  [unwired: 9 in, 1 out]
        n276 = Greater?(x=w228, y=u32 2000) -> (0:→"Battery_Critical":bool)
        n277 = local read "Dashboard Tab"() -> (w358:T1)
        n278 = call-poly <vilib>:"NT Read Value.vi"("Name"="Range_Right") -> ("Numeric"=→"Range_Right":dbl)  [unwired: 9 in, 1 out]
        n279 = call-poly <vilib>:"NT Read Value.vi"("Name"="Tank_Pressure") -> ("Numeric"=→"Tank_Pressure" →"Pressure_Visualize":dbl)  [unwired: 9 in, 1 out]
        n280 = call-poly <vilib>:"NT Read Value.vi"("Name"="Left_Drive_Vel") -> ("Numeric"=→"Left_Drive_Vel":dbl)  [unwired: 9 in, 1 out]
        n281 = call-poly <vilib>:"NT Read Value.vi"("Name"="Range_Front-Right") -> ("Numeric"=→"Range_Front-Right":dbl)  [unwired: 9 in, 1 out]
        n282 = call-poly <vilib>:"NT Read Value.vi"("Name"="Left_Drive_Pos") -> ("Numeric"=→"Left_Drive_Pos":dbl)  [unwired: 9 in, 1 out]
        n283 = call-poly <vilib>:"NT Read Value.vi"("Name"="Right_Drive_Pos") -> ("Numeric"=→"Right_Drive_Pos":dbl)  [unwired: 9 in, 1 out]
        n284 = call-poly <vilib>:"NT Read Value.vi"("Name"="Elevator_Power") -> ("Numeric"=→"Elevator_Power":dbl)  [unwired: 9 in, 1 out]
        n285 = To Double Precision Float(number="Climb_Level") -> (double precision float=w235:dbl)
        n286 = call-poly <vilib>:"NT Write Value.vi"("Boolean"="Overclock", "Name"="Overclock") -> ()  [unwired: 9 in, 1 out]
        n287 = call-poly <vilib>:"NT Read Value.vi"("Name"="Ground_Height") -> ("Numeric"=→"Ground_Height":dbl)  [unwired: 9 in, 1 out]
        n288 = Equal?(x=w358, y=T13."Tune") -> (x = y?=w356:bool)
        n289 = call-poly <vilib>:"NT Write Value.vi"("Boolean"="Defense_Driving", "Name"="Defense_Driving") -> ()  [unwired: 9 in, 1 out]
        n290 = call-poly <vilib>:"NT Write Value.vi"("Boolean"="LimeLight_Override", "Name"="LimeLight_Override") -> ()  [unwired: 9 in, 1 out]
        n291 = call-poly <vilib>:"NT Write Value.vi"("Numeric"=w235, "Name"="Climb_Level") -> ()  [unwired: 9 in, 1 out]
        n292 = call-poly <vilib>:"NT Write Value.vi"("Boolean"="Drive_Encoder_Reset", "Name"="Drive_Encoder_Reset") -> ()  [unwired: 9 in, 1 out]
        n293 = call-poly <vilib>:"NT Write Value.vi"("Boolean"=w356, "Name"="Tune_Tab") -> ()  [unwired: 9 in, 1 out]
      }
    }
  }
  n294 = control-ref of="Test Tree"() -> (w34:refnum<vi>)
  n295 = call "Initialize Camera and CheckList.vi"("ListBox in"=w20) -> ()  [unwired: 11 in]
  n296 = Index Array(array=w33) -> (element=w31:refnum<vi>)  [unwired: 1 in]
  n297 = vi-ref "Playback Controls.vi"() -> (w30:refnum<vi>)
  n298 = while {
    tunnel: w31 -> [w511]
    i -> [w514]
    stop <- FALSE stop-if-true
    n299 = Wait (ms)(milliseconds to wait=u32 100) -> ()  [unwired: 1 out]
    n300 = case shown="\"Playback\"" "Rec Mode" {
      tunnel: w514 -> [_ _ w529]
      tunnel: [u32 2829099 ("Base Color") u32 11141120 ("Target Color") w518] -> w510
      frame "Stop", Default {
        # "Reset the color, extra updates don't cost much"
      }
      frame "Record" {
      }
      frame "Playback" {
        # "Playback"
        n301 = Quotient & Remainder(x=w529, y=u32 50 ("milliseconds to wait")) -> (x-y*floor(x/y)=w525:u32)  [unwired: 1 out]
        n302 = Divide(x=w525, y=u32 50 ("milliseconds to wait")) -> (x/y=w522:dbl)
        n303 = Multiply(x=6.283185307179586, y=w522) -> (x*y=w527:dbl)
        n304 = Sine(x=w527) -> (sin(x)=w526:dbl)
        n305 = Absolute Value(x=w526) -> (abs(x)=w519:dbl)
        n306 = call "Interpolate RGB Color.vi"("Proportion"=w519, "Target Color"=u32 30976, "Base Color"=u32 2829099) -> ("Result Color"=w518:u32)  [unwired: 8 in]
      }
    }
    n307 = property class="Pane"(reference=w511, "PaneColor"=w510) -> ()  [unwired: 1 in, 2 out]
  }
  n308 = while {
    tunnel: [w539] -> _
    tunnel: w34 -> [w538]
    tunnel: w30 -> [w537]
    tunnel: w29 -> [w536]
    tunnel: w28 -> [_]
    tunnel: w24 -> [w535]
    tunnel: w12 -> [w534]
    tunnel: w11 -> [w533]
    shift-right: [w532] -> _
    shift-left: _ -> [w531]
    tunnel: w9 -> [w530]
    i -> [w539]
    stop <- FALSE stop-if-true
    n309 = event shown="[0] Timeout" {
      selector: w536 -> [_ _ _ _ _ _ _ _ _ _ _ _ _ _ _ _ _ _ _ _ _]
      dyn-events: [_ _ _ _ _ _ _ _ _ _ _ _ _ _ _ _ w797 _ _ _ _] -> _
      timeout: u32 60 ("milliseconds to wait") -> [_ _ _ _ _ _ _ _ _ _ _ _ _ _ _ _ _ _ _ _ _]
      tunnel: w538 -> [w551 _ _ _ _ _ _ _ _ _ _ _ _ _ _ _ _ _ _ _ _]
      tunnel: "Test Tree" -> [_ _ _ _ _ _ _ _ _ _ _ w766 w774 w776 w780 w788 _ _ _ _ _]
      tunnel: w537 -> [_ _ _ _ _ _ _ _ _ _ _ _ _ _ _ _ w799 _ w817 _ _]
      tunnel: w535 -> [_ _ _ _ _ _ _ _ _ _ _ _ _ _ _ _ w795 _ _ _ _]
      tunnel: w534 -> [_ _ _ _ _ _ _ _ _ _ _ _ _ _ _ _ w793 _ _ _ _]
      tunnel: w533 -> [w546 _ _ _ _ _ w717 _ _ _ _ _ _ _ _ _ _ _ _ _ _]
      tunnel: [w545 w594 w696 w701 w710 w714 w715 w724 w734 w741 w753 w765 w772 w775 w779 w787 w792 w812 w814 w818 w831] -> w532
      tunnel: w531 -> [w545 w594 w696 w701 w710 w714 w715 _ _ w741 w753 w765 w772 w775 w779 w787 w792 w812 w814 w818 w831]
      tunnel: w530 -> [w543 _ _ _ _ _ _ _ _ _ _ _ _ _ _ _ _ _ _ _ _]
      event Timeout {
        n310 = event-data() -> ()  [unwired: 1 in, 1 out]
        n311 = local read "Mode"() -> (w548:T5)
        n312 = case shown="\"Commands\"" "Dashboard Tab" {
          tunnel: w551 -> [_ _ w567 _ _]
          tunnel: "TestMode/Automatic/" ("Name Pattern") -> [_ _ w566 _ _]
          tunnel: T18 [{"Operation"=enum."Clear", "Color Box"=14013909}, {"Operation"=enum."Clear", "Color Box"=14013909}, {"Operation"=enum."Clear", "Color Box"=14013909}, {"Operation"=enum."Clear", "Color Box"=14013909}, {"Operation"=enum."Update", "Color Box"=14013909}, {"Operation"=enum."Update", "Color Box"=16777215}, {"Operation"=enum."Clear", "Color Box"=14013909}, {"Operation"=enum."Clear", "Color Box"=14013909}, {"Operation"=enum."Clear", "Color Box"=14013909}] -> [_ _ w559 _ w587]
          tunnel: w548 -> [_ _ w558 _ w586]
          tunnel: u32[] [15790320, 15790320, 15790320, 15790320, 16777215, 16777215, 15790320, 15790320, 15790320] -> [_ _ _ _ w592]
          tunnel: w546 -> [_ _ _ _ w580]
          tunnel: w543 -> [_ w553 _ _ _]
          frame "TeleOp", Default {
          }
          frame "Tune" {
            n313 = call <vilib>:"WPI_DashboardUpdateNames.vi"("Controls on Tab"=w553) -> ()  [unwired: 11 in]
          }
          frame "Test" {
            w565 = -2 ("Active Item:Row Number")
            n314 = Index Array(array=w559, index=w558) -> (element=w560:T21)
            n315 = Unbundle(w560) -> ("Operation"=w561:enum16{"Update", "Clear"}, "Color Box"=w562:u32)
            n316 = call <vilib>:"NT Read String.vi"("Name"="TestMode/TestName") -> ("String"=w556:string)  [unwired: 9 in, 1 out]
            n317 = call <vilib>:"NT Read and Format Entries as Tree.vi"("Operation"=w561, "Name Pattern"=w566, "Tree Refnum"=w567) -> ()  [unwired: 7 in, 2 out]
            n318 = case shown="\"\"" w556 {
              tunnel: "TestMode/TestProgress" ("Name") -> [w569 _]
              tunnel: "TestMode/TestProgressText" ("Name") -> [w568 _]
              frame Default {
                n319 = call <vilib>:"NT Read Number.vi"("Name"=w569) -> ("Numeric"=w570:dbl)  [unwired: 9 in, 1 out]
                n320 = call <vilib>:"NT Read String.vi"("Name"=w568) -> ("String"=w571:string)  [unwired: 9 in, 1 out]
                n321 = Bundle("Numeric"=w570, "String"=w571) -> (→"Progress":cluster{"Numeric":dbl, "String":string})  [unwired: 1 in]
              }
              frame "" {
                n322 = property on="Progress" class="Clust (strict)"("Visible"=FALSE) -> ()  [unwired: 2 in, 2 out]
                n323 = local write "Test Name"(u16 0) -> ()
              }
            }
            n324 = property on="Test Tree" class="Tree (strict)"("Active Item Row Number"=w565, "ActiveColNum"=w565, "CellBG"=w562, "Active Item Row Number"=-1 ("Active Item:Row Number"), "CellBG"=u32 5789784 ("Color Box")) -> ()  [unwired: 2 in, 2 out]
          }
          frame "Variables" {
            w577 = string[] ["CameraPublisher", "Usage", "DB"]  # Items to initially close
            n325 = First Call?() -> (First Call?: T/F=w578:bool)
            n326 = control-ref of="Tree"() -> (w579:refnum<vi>)
            n327 = Select(t=w577, s=w578, f=string[] []) -> (s? t:f=w575:string[])
            n328 = call <vilib>:"NT Read and Format Entries as Tree.vi"("Tags to  Close"=w575, "Tree Refnum"=w579) -> ()  [unwired: 8 in, 2 out]
          }
          frame "Commands" {
            w588 = u32 5789784 ("Color Box")
            w589 = T22 {"Row"=-1, "Column"=-2} ("Active Cell:Active Cell")
            w591 = T22 {"Row"=-2, "Column"=-2} ("Active Cell:Active Cell")
            n329 = Index Array(array=w592, index=w586) -> (element=w590:u32)
            n330 = Index Array(array=w587, index=w586) -> (element=w585:T21)
            n331 = Unbundle(w585) -> ("Operation"=w584:enum16{"Update", "Clear"})  [unwired: 1 out]
            n332 = local read "Command Selection"() -> (w583:i32)
            n333 = property on="Command Selection" class="MCListbox (strict)"("ActiveCell"=w591, "CellBG"=w590, "ActiveCell"=w589, "CellBG"=w588) -> ()  [unwired: 2 in, 2 out]
            n334 = call <vilib>:"WPI_DashboardUpdate RPC Info.vi"("Operation"=w584) -> ("update"=w582:bool, "commands"=w581:string[][])  [unwired: 9 in]
            n335 = property on="Command Selection" class="MCListbox (strict)"("ItemNames"=w581) -> ()  [unwired: 2 in, 2 out]
            n336 = property on="Command Params" class="Tbl (strict)"("Active Cell"=w591, "Cell BG Color"=w590, "Active Cell"=w589, "Cell BG Color"=w588) -> ()  [unwired: 2 in, 2 out]
            n337 = call <vilib>:"WPI_DashboardUpdate Command Params.vi"("Update"=w582, "NewVal"=w583, "Commands"=w581, "Param Tbl"=w580) -> ()  [unwired: 7 in, 1 out]
          }
        }
        n338 = call <vilib>:"Connextion Info.vi"() -> ("Connected"=→"NT Connection":bool)  [unwired: 10 in, 1 out]
      }
      event "Test Tree": Value Change {
        # "Show appropriate\ncontrols"
        n339 = event-data() -> ("CtlRef"=w597:refnum<vi>, "NewVal"=w595:string)  [unwired: 1 in]
        n340 = call <vilib>:"WPI_UtilitiesGetTreeIOName.vi"("NewVal"=w595, "TreeControl in"=w597) -> ("I/O Name"=w598:string)  [unwired: 9 in]
        n341 = case shown="\"Analog Out\", \"Motor\", \"PWM\"" w598 {
          selector: w598 -> [_ w605 _ w627 w636 _]
          tunnel: w595 -> [_ _ w624 w626 _ w643]
          tunnel: cluster{string[]}[] [{["640x480", "320x240", "160x120"]}, {["Auto", "Fixed indoor", "Fixed outdoor 1", "Fixed outdoor 2", "Fixed fluorescent 1", "Fixed fluorescent 2", "Hold current"]}, {["Auto", "Flicker-free 50 Hz", "Flicker-free 60 Hz", "Hold current"]}, {["None", "Prioritize frame rate", "Prioritize image quality"]}, {["Monochrome", "Color"]}] -> [_ _ _ _ _ w642]
          frame Default {
            w600 = FALSE ("Visible")
            w599 = FALSE ("Visible")
            n342 = property on="Motor" class="Clust (strict)"("Visible"=w599) -> ()  [unwired: 2 in, 2 out]
            n343 = property on="Test Ring" class="Ring (strict)"("Visible"=w599) -> ()  [unwired: 2 in, 2 out]
            n344 = property on="Rev/Fwd" class="Clust (strict)"("Visible"=w600) -> ()  [unwired: 2 in, 2 out]
            n345 = property on="On/Off" class="Bool (strict)"("Visible"=w600) -> ()  [unwired: 2 in, 2 out]
            n346 = property on="Test Slider" class="Slide (strict)"("Visible"=w600) -> ()  [unwired: 2 in, 2 out]
          }
          frame "Analog Out", "Motor", "PWM" {
            w606 = FALSE ("Visible")
            n347 = case shown="\"Analog Out\"" w605 {
              tunnel: [1.0 ("Value") -1.0 ("Value") 0.0 ("Value")] -> w604
              tunnel: [255.0 ("Value") 1.0 ("Value") 5.0 ("Value")] -> w603
              tunnel: [128.0 ("Value") 0.0 ("Value") 0.0 ("Value")] -> w602
              tunnel: [64.0 ("Value") 0.5 ("Value") 1.0 ("Value")] -> w601
              frame "PWM" {
              }
              frame "Motor", Default {
              }
              frame "Analog Out" {
              }
            }
            n348 = property on="Motor" class="Clust (strict)"("Visible"=TRUE) -> ()  [unwired: 2 in, 2 out]
            n349 = property on="Value" class="Slide (strict)"("Value"=w602, "Scale.Minimum"=w604, "Scale.Maximum"=w603, "Scale.Increment"=w601) -> ()  [unwired: 2 in, 2 out]
            n350 = property on="On/Off" class="Bool (strict)"("Visible"=w606) -> ()  [unwired: 2 in, 2 out]
            n351 = property on="Test Slider" class="Slide (strict)"("Visible"=w606) -> ()  [unwired: 2 in, 2 out]
            n352 = property on="Test Ring" class="Ring (strict)"("Visible"=w606) -> ()  [unwired: 2 in, 2 out]
            n353 = property on="Rev/Fwd" class="Clust (strict)"("Visible"=w606) -> ()  [unwired: 2 in, 2 out]
          }
          frame "Servo" {
            w622 = FALSE ("Visible")
            n354 = call <vilib>:"NT Read Number.vi"("Name"=w624) -> ("Numeric"=w623:dbl)  [unwired: 9 in, 1 out]
            n355 = property on="Test Slider" class="Slide (strict)"("Visible"=TRUE, "Scale.Maximum"=170.0 ("Scale.Range:Maximum")) -> ()  [unwired: 2 in, 2 out]
            n356 = local write "Test Slider"(w623) -> ()
            n357 = property on="Motor" class="Clust (strict)"("Visible"=w622) -> ()  [unwired: 2 in, 2 out]
            n358 = property on="Rev/Fwd" class="Clust (strict)"("Visible"=w622) -> ()  [unwired: 2 in, 2 out]
            n359 = property on="On/Off" class="Bool (strict)"("Visible"=w622) -> ()  [unwired: 2 in, 2 out]
            n360 = property on="Test Ring" class="Ring (strict)"("Visible"=w622) -> ()  [unwired: 2 in, 2 out]
          }
          frame "Relay", "Solenoid" {
            w625 = FALSE ("Visible")
            n361 = property on="Motor" class="Clust (strict)"("Visible"=w625) -> ()  [unwired: 2 in, 2 out]
            n362 = property on="Test Slider" class="Slide (strict)"("Visible"=w625) -> ()  [unwired: 2 in, 2 out]
            n363 = Search and Replace String(input string=w626, search string="/Value  **", replace string="/Direction") -> (result string=w632:string)  [unwired: 5 in, 3 out]
            n364 = property on="Test Ring" class="Ring (strict)"("Visible"=w625) -> ()  [unwired: 2 in, 2 out]
            n365 = call <vilib>:"NT Read String.vi"("Name"=w632) -> ("String"=w630:string)  [unwired: 9 in, 1 out]
            n366 = Equal?(x="Both directions", y=w630) -> (x = y?=w628:bool)
            n367 = Not(x=w628) -> (.not. x?=w629:bool)
            n368 = property on="Rev/Fwd" class="Clust (strict)"("Visible"=w628) -> ()  [unwired: 2 in, 2 out]
            n369 = property on="On/Off" class="Bool (strict)"("Visible"=w629, "Caption.Text"=w627) -> ()  [unwired: 2 in, 2 out]
          }
          frame "Compressor", "Digital Out" {
            w635 = FALSE ("Visible")
            # "Get direction and finish"
            n370 = property on="Motor" class="Clust (strict)"("Visible"=w635) -> ()  [unwired: 2 in, 2 out]
            n371 = property on="Test Slider" class="Slide (strict)"("Visible"=w635) -> ()  [unwired: 2 in, 2 out]
            n372 = property on="Test Ring" class="Ring (strict)"("Visible"=w635) -> ()  [unwired: 2 in, 2 out]
            n373 = property on="On/Off" class="Bool (strict)"("Visible"=TRUE, "Caption.Text"=w636) -> ()  [unwired: 2 in, 2 out]
            n374 = property on="Rev/Fwd" class="Clust (strict)"("Visible"=FALSE) -> ()  [unwired: 2 in, 2 out]
          }
          frame "Camera" {
            n375 = call <vilib>:"Get Last Path Segment.vi"("String in"=w643) -> ("String out"=w644:string)  [unwired: 10 in]
            n376 = property on="On/Off" class="Bool (strict)"("Visible"=FALSE) -> ()  [unwired: 2 in, 2 out]
            n377 = property on="Motor" class="Clust (strict)"("Visible"=FALSE) -> ()  [unwired: 2 in, 2 out]
            n378 = property on="Rev/Fwd" class="Clust (strict)"("Visible"=FALSE) -> ()  [unwired: 2 in, 2 out]
            n379 = case shown="\"White Balance  **\"" w644 {
              tunnel: w643 -> [w650 w659 w668 w677 w686 _ w692]
              tunnel: w642 -> [w648 w656 w665 w674 w683 _ _]
              frame "Size  **" {
                n380 = Index Array(array=w648) -> (element=w647:cluster{string[]})  [unwired: 1 in]
                n381 = call <vilib>:"NT Read String.vi"("Name"=w650) -> ("String"=w649:string)  [unwired: 9 in, 1 out]
                n382 = Unbundle(w647) -> (w645:string[])
                n383 = Match First String(2:w645, 3:w649) -> (0:w646:i32)  [unwired: 1 out]
                n384 = property on="Test Ring" class="Ring (strict)"("Value"=w646, "Strings []"=w645) -> ()  [unwired: 2 in, 2 out]
                n385 = property on="Test Ring" class="Ring (strict)"("Visible"=TRUE) -> ()  [unwired: 2 in, 2 out]
                n386 = property on="Test Slider" class="Slide (strict)"("Visible"=FALSE) -> ()  [unwired: 2 in, 2 out]
              }
              frame "White Balance  **" {
                n387 = Index Array(array=w656, index=1) -> (element=w657:cluster{string[]})
                n388 = call <vilib>:"NT Read String.vi"("Name"=w659) -> ("String"=w658:string)  [unwired: 9 in, 1 out]
                n389 = Unbundle(w657) -> (w654:string[])
                n390 = Match First String(2:w654, 3:w658) -> (0:w653:i32)  [unwired: 1 out]
                n391 = property on="Test Ring" class="Ring (strict)"("Value"=w653, "Strings []"=w654) -> ()  [unwired: 2 in, 2 out]
                n392 = property on="Test Ring" class="Ring (strict)"("Visible"=TRUE) -> ()  [unwired: 2 in, 2 out]
                n393 = property on="Test Slider" class="Slide (strict)"("Visible"=FALSE) -> ()  [unwired: 2 in, 2 out]
              }
              frame "Exposure  **" {
                n394 = Index Array(array=w665, index=2) -> (element=w666:cluster{string[]})
                n395 = call <vilib>:"NT Read String.vi"("Name"=w668) -> ("String"=w667:string)  [unwired: 9 in, 1 out]
                n396 = Unbundle(w666) -> (w662:string[])
                n397 = Match First String(2:w662, 3:w667) -> (0:w663:i32)  [unwired: 1 out]
                n398 = property on="Test Ring" class="Ring (strict)"("Value"=w663, "Strings []"=w662) -> ()  [unwired: 2 in, 2 out]
                n399 = property on="Test Ring" class="Ring (strict)"("Visible"=TRUE) -> ()  [unwired: 2 in, 2 out]
                n400 = property on="Test Slider" class="Slide (strict)"("Visible"=FALSE) -> ()  [unwired: 2 in, 2 out]
              }
              frame "Exposure Priority  **" {
                n401 = Index Array(array=w674, index=3) -> (element=w675:cluster{string[]})
                n402 = call <vilib>:"NT Read String.vi"("Name"=w677) -> ("String"=w676:string)  [unwired: 9 in, 1 out]
                n403 = Unbundle(w675) -> (w671:string[])
                n404 = Match First String(2:w671, 3:w676) -> (0:w672:i32)  [unwired: 1 out]
                n405 = property on="Test Ring" class="Ring (strict)"("Value"=w672, "Strings []"=w671) -> ()  [unwired: 2 in, 2 out]
                n406 = property on="Test Ring" class="Ring (strict)"("Visible"=TRUE) -> ()  [unwired: 2 in, 2 out]
                n407 = property on="Test Slider" class="Slide (strict)"("Visible"=FALSE) -> ()  [unwired: 2 in, 2 out]
              }
              frame "Color Enable  **" {
                n408 = Index Array(array=w683, index=4) -> (element=w684:cluster{string[]})
                n409 = call <vilib>:"NT Read String.vi"("Name"=w686) -> ("String"=w685:string)  [unwired: 9 in, 1 out]
                n410 = Unbundle(w684) -> (w680:string[])
                n411 = Match First String(2:w680, 3:w685) -> (0:w681:i32)  [unwired: 1 out]
                n412 = property on="Test Ring" class="Ring (strict)"("Value"=w681, "Strings []"=w680) -> ()  [unwired: 2 in, 2 out]
                n413 = property on="Test Ring" class="Ring (strict)"("Visible"=TRUE) -> ()  [unwired: 2 in, 2 out]
                n414 = property on="Test Slider" class="Slide (strict)"("Visible"=FALSE) -> ()  [unwired: 2 in, 2 out]
              }
              frame Default {
                n415 = property on="Test Ring" class="Ring (strict)"("Visible"=FALSE) -> ()  [unwired: 2 in, 2 out]
                n416 = property on="Test Slider" class="Slide (strict)"("Visible"=FALSE) -> ()  [unwired: 2 in, 2 out]
              }
              frame "Brightness  **", "Color Level  **", "Compression  **", "FPS  **", "Sharpness  **" {
                n417 = call <vilib>:"NT Read Number.vi"("Name"=w692) -> ("Numeric"=w691:dbl)  [unwired: 9 in, 1 out]
                n418 = local write "Test Slider"(w691) -> ()
                n419 = property on="Test Slider" class="Slide (strict)"("Visible"=TRUE, "Scale.Maximum"=100.0 ("Scale.Range:Maximum")) -> ()  [unwired: 2 in, 2 out]
                n420 = property on="Test Ring" class="Ring (strict)"("Visible"=FALSE) -> ()  [unwired: 2 in, 2 out]
              }
            }
          }
        }
        n421 = property on="Progress" class="Clust (strict)"("Visible"=FALSE) -> ()  [unwired: 2 in, 2 out]
      }
      event "Test Name": Mouse Enter {
        # "Populate the ring with the list of tests"
        n422 = event-data() -> ()  [unwired: 1 in, 1 out]
        n423 = call <vilib>:"NT Read String Array.vi"("Name"="TestMode/TestList") -> ("String Array"=w700:string[])  [unwired: 9 in, 1 out]
        n424 = Build Array (concatenate)("Select the test to run...", w700) -> (w699:string[])
        n425 = property on="Test Name" class="Ring (strict)"("Strings []"=w699) -> ()  [unwired: 2 in, 2 out]
      }
      event "Test Name": Value Change {
        w702 = FALSE ("Visible")
        # "Tell the robot the test name to run"
        n426 = event-data() -> ("NewVal"=w706:u16)  [unwired: 1 in]
        n427 = property on="Test Name" class="Ring (strict)"() -> ("Strings []"=w707:string[])  [unwired: 2 in, 2 out]
        n428 = local write "Progress"(T6 {"Test Progress"=0, "Test Progress Text"=""} ("Progress")) -> ()
        n429 = Index Array(array=w707, index=w706) -> (element=w705:string)
        n430 = call <vilib>:"NT Write String.vi"("String"=w705, "Name"="TestMode/TestName") -> ()  [unwired: 9 in, 1 out]
        n431 = property on="Progress" class="Clust (strict)"("Visible"=TRUE) -> ()  [unwired: 2 in, 2 out]
        n432 = property on="Motor" class="Clust (strict)"("Visible"=w702) -> ()  [unwired: 2 in, 2 out]
        n433 = property on="Test Slider" class="Slide (strict)"("Visible"=w702) -> ()  [unwired: 2 in, 2 out]
        n434 = property on="On/Off" class="Bool (strict)"("Visible"=w702) -> ()  [unwired: 2 in, 2 out]
        n435 = property on="Rev/Fwd" class="Clust (strict)"("Visible"=w702) -> ()  [unwired: 2 in, 2 out]
        n436 = property on="Test Ring" class="Ring (strict)"("Visible"=w702) -> ()  [unwired: 2 in, 2 out]
      }
      event "Select Auto": Mouse Enter {
        # "Populate the combo box with the list of autonomous options"
        n437 = event-data() -> ()  [unwired: 1 in, 1 out]
        n438 = call <vilib>:"NT Read String Array.vi"("Name"="Auto List") -> ("String Array"=w709:string[])  [unwired: 9 in, 1 out]
        n439 = property on="Select Auto" class="CmbBox"("Strings[]"=w709) -> ()  [unwired: 2 in, 2 out]
      }
      event "Select Auto": Value Change {
        # "User modified the Auto Selection. Write to NT variable so robot knows."
        n440 = event-data() -> ("NewVal"=w712:string)  [unwired: 1 in]
        n441 = call <vilib>:"NT Write String.vi"("String"=w712, "Name"="Auto Selector") -> ()  [unwired: 9 in, 1 out]
      }
      event "Command Selection": Value Change {
        # "Get the params and show in table"
        n442 = event-data() -> ("NewVal"=w718:i32)  [unwired: 1 in]
        n443 = property on="Command Selection" class="MCListbox (strict)"() -> ("ItemNames"=w716:string[][])  [unwired: 2 in, 2 out]
        n444 = call <vilib>:"WPI_DashboardUpdate Command Params.vi"("NewVal"=w718, "Commands"=w716, "Param Tbl"=w717) -> ()  [unwired: 8 in, 1 out]
      }
      event "Execute Command": Value Change {
        # "Started one, Unique ID holds\nresponse"
        n445 = event-data() -> ()  [unwired: 1 in, 1 out]
        n446 = property on="Command Selection" class="MCListbox (strict)"() -> ("ItemNames"=w729:string[][])  [unwired: 2 in, 2 out]
        n447 = Index Array(array=w729, index (row)="Command Selection", index (col)=0) -> (element=w727:string)
        n448 = call <vilib>:"Invoke Commands.vi"("Command Params"="Command Params", "Function Name"=w727) -> ("Params"=w723:u8, "Started"=w722:bool)  [unwired: 7 in, 1 out]
        n449 = Array Subset(array="Command Params", length (row)=w723) -> (w724:string[][])  [unwired: 3 in]
        n450 = Select(t="Executing" ("Cmd Status"), s=w722, f="" ("Cmd Status")) -> (s? t:f=→"Cmd Status":string)
      }
      event "Command Selection": Double Click {
        n451 = event-data() -> ("Row"=w737:i32)  [unwired: 1 in]
        n452 = property on="Command Selection" class="MCListbox (strict)"() -> ("ItemNames"=w740:string[][])  [unwired: 2 in, 2 out]
        n453 = local read "Command Params"() -> (w736:string[][])
        n454 = Index Array(array=w740, index (row)=w737, index (col)=0) -> (element=w738:string)
        n455 = call <vilib>:"Invoke Commands.vi"("Command Params"=w736, "Function Name"=w738) -> ("Params"=w735:u8, "Started"=w730:bool)  [unwired: 7 in, 1 out]
        n456 = Array Subset(array=w736, length (row)=w735) -> (w734:string[][])  [unwired: 3 in]
        n457 = Select(t="Executing" ("Cmd Status"), s=w730, f="" ("Cmd Status")) -> (s? t:f=w731:string)
        n458 = local write "Cmd Status"(w731) -> ()
      }
      event "CheckList": Double Click {
        # "Shift clears all"
        # "Update symbols on the listbox"
        n459 = event-data() -> ("PlatMods.Shift"=w742:bool, "Row"=w744:i32)  [unwired: 1 in]
        n460 = case shown="True" w742 {
          tunnel: w744 -> [w748 _]
          tunnel: 1 -> [w747 _]
          frame False {
            n461 = property on="CheckList" class="LstBox (strict)"() -> ("Item Symbols"=w746:i32[])  [unwired: 2 in, 2 out]
            n462 = Replace Array Subset(array=w746, new element=w747, index=w748) -> (w745:i32[])
            n463 = property on="CheckList" class="LstBox (strict)"("Item Symbols"=w745) -> ()  [unwired: 2 in, 2 out]
          }
          frame True {
            w749 = 0 ("Top Row")
            n464 = property on="CheckList" class="LstBox (strict)"() -> ("Number of Rows"=w751:u32)  [unwired: 2 in, 2 out]
            n465 = Initialize Array(0, w751) -> (w750:i32[])
            n466 = property on="CheckList" class="LstBox (strict)"("Top Row"=w749, "Value"=w749, "Item Symbols"=w750) -> ()  [unwired: 2 in, 2 out]
          }
        }
      }
      event "CheckList": Key Down {
        # "Update symbols on the listbox\nLeft and right keys check and uncheck"
        n467 = event-data() -> ("VKey"=w755:T19)  [unwired: 1 in]
        n468 = case shown="\"Left\", \"Right\"" w755 {
          selector: w755 -> [w760 _]
          tunnel: eventvkey."Left" ("VKey") -> [w758 _]
          frame "Left", "Right" {
            n469 = Equal?(x=w758, y=w760) -> (x = y?=w759:bool)
            n470 = Select(t=0, s=w759, f=1) -> (s? t:f=w761:i32)
            n471 = property on="CheckList" class="LstBox (strict)"() -> ("Item Symbols"=w764:i32[])  [unwired: 2 in, 2 out]
            n472 = Replace Array Subset(array=w764, new element=w761, index="CheckList") -> (w763:i32[])
            n473 = property on="CheckList" class="LstBox (strict)"("Item Symbols"=w763) -> ()  [unwired: 2 in, 2 out]
          }
          frame Default {
          }
        }
      }
      event "Motor.Enable": Value Change {
        # "When the test mode otor enable helper is set, update that\ntree row item's value"
        n474 = event-data() -> ("NewVal"=w770:bool)  [unwired: 1 in]
        n475 = Unbundle("Motor") -> ("Value"=w769:dbl)  [unwired: 1 out]
        n476 = Select(t=w769, s=w770, f=0.0) -> (s? t:f=w767:dbl)
        n477 = call <vilib>:"NT Write Number.vi"("Numeric"=w767, "Name"=w766) -> ()  [unwired: 9 in, 1 out]
      }
      event "Test Slider": Value Change {
        # "When the test mode slider helper is set, update that\ntree row item's value"
        n478 = event-data() -> ("NewVal"=w773:dbl)  [unwired: 1 in]
        n479 = call <vilib>:"NT Write Number.vi"("Numeric"=w773, "Name"=w774) -> ()  [unwired: 9 in, 1 out]
      }
      event "On/Off": Value Change {
        # "When the test mode on/off helper value is set, update that\ntree row item's value"
        n480 = event-data() -> ("NewVal"=w778:bool)  [unwired: 1 in]
        n481 = Boolean To (0,1)(Boolean=w778) -> (0, 1=w777:i16)
        n482 = call <vilib>:"NT Write Number.vi"("Numeric"=w777, "Name"=w776) -> ()  [unwired: 9 in, 1 out]
      }
      event "Rev/Fwd": Value Change {
        # "When the test mode helper value for relays is set, update that\ntree row item's value"
        n483 = event-data() -> ("NewVal.Forward"=w786:bool, "NewVal.Reverse"=w785:bool)  [unwired: 1 in]
        n484 = Boolean To (0,1)(Boolean=w786) -> (0, 1=w782:i16)
        n485 = Boolean To (0,1)(Boolean=w785) -> (0, 1=w784:i16)
        n486 = Negate(x=w784) -> (-x=w783:i16)
        n487 = Add(x=w782, y=w783) -> (x+y=w781:i16)
        n488 = call <vilib>:"NT Write Number.vi"("Numeric"=w781, "Name"=w780) -> ()  [unwired: 9 in, 1 out]
      }
      event "Test Ring": Value Change {
        # "When a test mode helper value is selected from the ring,\nset the tree item's variable to the string value"
        n489 = event-data() -> ("NewVal"=w790:u16)  [unwired: 1 in]
        n490 = property on="Test Ring" class="Ring (strict)"() -> ("Strings []"=w791:string[])  [unwired: 2 in, 2 out]
        n491 = Index Array(array=w791, index=w790) -> (element=w789:string)
        n492 = call <vilib>:"NT Write String.vi"("String"=w789, "Name"=w788) -> ()  [unwired: 9 in, 1 out]
      }
      event "Rec Mode": Value Change {
        # "Update globals for recording mode and path to read log from.\nClear when logging and let NetworkTables set path for vision to\nuse."
        n493 = event-data() -> ("NewVal"=w800:enum32{"Stop", "Record", "Playback"})  [unwired: 1 in]
        n494 = global write "WPI_DashboardLogging Global.vi" "Logging Filename"(path "") -> ()
        n495 = global write "WPI_DashboardLogging Global.vi" "Recording"(w800) -> ()
        n496 = case shown="\"Playback\"" w800 {
          tunnel: w799 -> [_ w802 w811]
          tunnel: [_ _ w810] -> w797
          tunnel: [_ _ w809] -> _
          tunnel: w795 -> [_ _ w807]
          tunnel: cluster{i32, i32} {-250, 170} -> [_ _ w806]
          tunnel: [_ _ T20 {"Image Size"=TRUE, "Image Type"=TRUE, "Pixel Value"=TRUE, "ROI Information"=TRUE, "Zoom Factor"=FALSE} ("Image Information Shown:All Elements")] -> _
          tunnel: [_ _ TRUE ("Zoom Factor")] -> _
          tunnel: w793 -> [_ _ w803]
          frame Default {
          }
          frame "Stop", "Record" {
            # "Place Window too"
            n497 = invoke class="VI" method="FP.Close"(reference=w802) -> (reference out=w801:refnum<vi>)  [unwired: 2 in, 2 out]
            n498 = invoke class="VI" method="Abort VI"(reference=w801) -> ()  [unwired: 2 in, 3 out]
          }
          frame "Playback" {
            n499 = call "Open Playback Panel.vi"("Offset"=w806, "DB VI Ref"=w807, "Playback in"=w811) -> ("Playback out"=w808:refnum<vi>)  [unwired: 8 in]
            n500 = register-events(w808, w803) -> (reference out=w810:refnum<event-registration>, error out=w809:errorcluster)  [unwired: 2 in]
          }
        }
        n501 = call <vilib>:"WPI_DashboardNT Log FieldName Cache.vi"("Operation"=enum16{"Lookup/Add", "Index", "Clear"}."Clear") -> ()  [unwired: 8 in, 3 out]
      }
      event Panel Close {
        w813 = enum32{"Stop", "Record", "Playback"}."Stop" ("Rec Mode")
        # "Playback window has been closed, abort"
        n502 = event-data() -> ()  [unwired: 1 in, 4 out]
        n503 = local write "Rec Mode"(w813) -> ()
        n504 = global write "WPI_DashboardLogging Global.vi" "Recording"(w813) -> ()
      }
      event Panel Close {
        # "Abort playback window and ourself"
        n505 = event-data() -> ()  [unwired: 1 in, 4 out]
        n506 = invoke class="VI" method="FP.Close"(reference=w817) -> (reference out=w816:refnum<vi>)  [unwired: 2 in, 2 out]
        n507 = invoke class="VI" method="Abort VI"(reference=w816) -> (error out=w815:errorcluster)  [unwired: 2 in, 2 out]
        n508 = invoke class="VI" method="Abort VI"(error in=w815) -> ()  [unwired: 2 in, 3 out]
      }
      event User Event {
        n509 = event-data() -> ("IDs"=w824:cluster{"RPC field ID":u16, "Unique ID":u16}, "String"=w823:string)  [unwired: 1 in]
        n510 = Bundle("IDs"=w824, "String"=w823) -> (w822:T9)  [unwired: 1 in]
        n511 = call <vilib>:"Retrieve RPC Response.vi"("RPC Response"=w822) -> ("Output"=w820:string[][])  [unwired: 10 in]
        n512 = Build Array (concatenate)(w818, w820) -> (w819:string[][])
        n513 = local write "Command Params"(w819) -> ()
        n514 = local write "Cmd Status"("" ("Cmd Status")) -> ()
      }
      event "Tree": Double Click {
        n515 = event-data() -> ("PlatMods"=w830:T23, "Tag"=w827:string)  [unwired: 1 in]
        n516 = Unbundle(w830) -> ("Shift"=w829:bool)  [unwired: 4 out]
        n517 = String Subset(string=w827, length (rest)=1 ("length (rest)")) -> (substring=w826:string)  [unwired: 1 in]
        n518 = Not(x=w829) -> (.not. x?=w828:bool)
        n519 = case shown="\"/\"" w826 {
          tunnel: w827 -> [_ w833]
          tunnel: w828 -> [_ w832]
          frame Default {
          }
          frame "/" {
            n520 = call <vilib>:"NT Update Persistence.vi"("Persistence"=w832, "Name"=w833) -> ()  [unwired: 9 in, 1 out]
          }
        }
      }
    }
  }
  n521 = while {
    tunnel: u16 1741 ("timeout ms (25000)") -> [w835]
    stop <- FALSE stop-if-true
    n522 = TCP Create Listener(10:w835) -> (0:w834:errorcluster, 3:w836:refnum<k5>)  [unwired: 4 in, 1 out]
    n523 = case shown="No Error" w834 {
      selector: w834 -> [w838 _]
      tunnel: w836 -> [w839 _]
      frame No Error {
        n524 = while {
          tunnel: w839 -> [w842]
          tunnel: w838 -> [w841]
          stop <- FALSE stop-if-true
          n525 = TCP Wait On Listener(8:w841, 11:w842) -> (0:w843:errorcluster, 4:w844:refnum<k5>)  [unwired: 2 in, 3 out]
          n526 = local write "TCP"(w844) -> ()
          n527 = case shown="No Error" w843 {
            frame No Error {
            }
            frame Error {
              n528 = Wait (ms)(milliseconds to wait=u32 1000) -> ()  [unwired: 1 out]
            }
          }
        }
      }
      frame Error {
        n529 = Wait (ms)(milliseconds to wait=u32 1000) -> ()  [unwired: 1 out]
      }
    }
  }
  n530 = local write "Dashboard Tab"(T1."Checklist" ("Dashboard Tab")) -> ()
  n531 = property on="On/Off" class="Bool (strict)"("Visible"=w19) -> ()  [unwired: 2 in, 2 out]
  n532 = property on="Motor" class="Clust (strict)"("Visible"=w19) -> ()  [unwired: 2 in, 2 out]
  n533 = property on="Progress" class="Clust (strict)"("Visible"=w19) -> ()  [unwired: 2 in, 2 out]
  n534 = property on="Test Ring" class="Ring (strict)"("Visible"=w19) -> ()  [unwired: 2 in, 2 out]
  n535 = property on="Rev/Fwd" class="Clust (strict)"("Visible"=w19) -> ()  [unwired: 2 in, 2 out]
  n536 = local write "Command Selection"(u16 0 ("milliseconds to wait")) -> ()
  n537 = local write "Command Params"(string[][] [] ("Command Params")) -> ()
  n538 = global write "WPI_DashboardLogging Global.vi" "Recording"(w25) -> ()
  n539 = local write "Rec Mode"(w25) -> ()
  n540 = call <vilib>:"NT Write String.vi"("String"="Select Auto", "Name"="Auto Selector") -> ()  [unwired: 9 in, 1 out]
  n541 = while {
    tunnel: w1 -> [_]
    stop <- FALSE stop-if-true
    # "Error Message Handling"
    n542 = local read "Tilt_Safety_Override"() -> (w883:bool)
    n543 = local read "Tilt_Interlock"() -> (w869:bool)
    n544 = local read "Super_Test_Mode"() -> (w885:bool)
    n545 = local read "Elevator_Manual"() -> (w884:bool)
    n546 = local read "Master_Safety_Override_1"() -> (w879:bool)
    n547 = local read "Master_Safety_Override_2"() -> (w880:bool)
    n548 = local read "Check_Limit_Switch"() -> (w875:bool)
    n549 = local read "Elevator_Stall"() -> (w872:bool)
    n550 = local read "E1 Warning"() -> (w866:bool)
    n551 = local read "E2 Warning"() -> (w865:bool)
    n552 = local read "E3 Warning"() -> (w864:bool)
    n553 = local read "State_Conflict"() -> (w857:bool)
    n554 = local read "Battery_Critical"() -> (w854:bool)
    n555 = local read "Pressure_Leak"() -> (w851:bool)
    n556 = And(x=w879, y=w880) -> (x .and. y?=w878:bool)
    n557 = Build Array(1000.0, 1000.0, 1000.0 ("element"), 1000.0 ("element"), 10.0 ("element"), 10.0 ("element"), 3.0 ("element"), 10.0 ("element"), 10.0 ("element"), 10.0 ("element"), 3.0 ("element"), 10.0 ("element"), 10.0 ("element")) -> (w887:dbl[])
    n558 = Build Array("super test mode", "elevator in manual mode", "tilt safety disabled" ("element"), "all safeties disabled" ("element"), "elevator limit switch failure" ("element"), "elevator is stalling" ("element"), "reset tilt interlock" ("element"), "elevator motor 1 has failed" ("element"), "elevator motor 2 has failed" ("element"), "elevator motor 3 has failed" ("element"), "eject game piece" ("element"), "battery low" ("element"), "pressure leak detected" ("element")) -> (w890:string[])
    n559 = Build Array(w885, w884, w883, w878, w875, w872, w869, w866, w865, w864, w857, w854, w851) -> (w847:bool[])
    n560 = call "ErrorMessageBuilder.vi"("Error Triggers"=w847, "Delays (s)"=w887, "Error Messages"=w890) -> ("Combined Error String"=w848:string)  [unwired: 2 in]
    "Combined Error String" <- w848
    n561 = call "TextToSpeech.vi"("Text To Be Spoken"=w848) -> ()  [unwired: 9 in, 2 out]
    n562 = Wait (ms)(milliseconds to wait=u32 200) -> ()  [unwired: 1 out]
  }
